vi "Tremor Interface.vi"() -> ()   [LabVIEW 2010]
uses:
  <vilib>/userDefined/High Color/IMAQdx.ctl
  Classes/Imported FFT Data.lvclass
  Controls/Interface states.ctl
  Classes/Waveform data.lvclass
  Classes/Video feed info.lvclass
  Controls/Timing Control.ctl
  Classes/Timer.lvclass
  <vilib>/Utility/xml.llb/Read From XML File(string).vi
  <vilib>/Analysis/2dsp.llb/1D Auto Correlation (DBL).vi
  <vilib>/Utility/xml.llb/Write to XML File(string).vi
  <vilib>/Utility/file.llb/Read From Spreadsheet File (string).vi
  <vilib>/Utility/file.llb/Read From Spreadsheet File (DBL).vi
  <vilib>/vision/NI_Vision_Development_Module.lvlib
  <vilib>/Analysis/NI_AAL_SigProc.lvlib
  <vilib>/Analysis/NI_AALBase.lvlib
  <vilib>/Analysis/NI_AALPro.lvlib
panel:
  in  "Reset spin":bool caption="Stop (F)"
  in  "spin control":bool caption="Stop (F)"
  in  "indicator radius":i16=10
  in  "indicator color":u32(colorbox)
  in  "speed":dbl=3.0
  in  "radius out":i16=130
  in  "camera feed":T1="cam0"
  in  "Circle width":i8(knob) scale=1.0..50.0
  in  "fill static indicator":bool
  in  "Circle style":T2(ring)
  in  "center color":u32(colorbox)
  in  "dot color":u32(colorbox)=782080
  out "Y Resolution":i32
  out "X Resolution":i32
  in  "Image Type":T3 items=["Grayscale (U8)", "Grayscale (I16)", "Grayscale (SGL)", "Complex (CSG)", "RGB (U32)", "HSL (U32)", "RGB (U64)", "Grayscale (U16)"]
  out "Frame Rate":dbl
  out "Image Number":u32
  in  "analyze (F3)":bool caption="Stop (F)"
  in  "record (F2)":bool caption="Stop (F)"
  in  "Save Config":bool caption="Stop (F)"
  in  "Optical FFTs":bool
  in  "Optical Data":bool
  out "number of channels":i32
  in  "Reset":bool caption="Stop (F)"
  in  "Quit":bool caption="Stop (F)"
  in  "camera (F1)":bool caption="Stop (F)"
  in  "Tab Control":T4(tab)
  out "Testing area":picture
  out "distance":dbl[](graph)
  out "distance":dbl
  out "angles":dbl[](graph)
  out "angles":dbl
  out "outside":bool
  out "Time outside circles":string
  out "outer counter":i8
  out "exterior":bool
  out "Time in exterior circle":string
  out "exterior counter":i8
  out "middle":bool
  out "Time in middle circle":string
  out "middle counter":i8
  out "interior":bool
  out "Time in inner circle":string
  out "inner counter":i8
  in  "Reset times":bool caption="Stop (F)"
  out "raw display":T5(plugin-control)
  in  "exterior color":u32(colorbox)=16711680
  in  "exterior circle":i16(knob)=164 scale=196.0..215.6
  in  "middle color":u32(colorbox)=16711680
  in  "middle circle":i16(knob)=93 scale=100.0..196.0
  in  "interior color":u32(colorbox)=16711680
  in  "interior circle":i16(knob)=57 scale=50.0..156.0
  in  "Rewind":bool
  in  "Forward":bool
  in  "Play/Stop":bool
  in  "Load file":bool
  in  "Video feed tab control":enum32{"Data", "Video controls"}(tab)
  out "displacement - vp":dbl[][](graph) caption="displacement"
  out "angles - vp":dbl[][](graph) caption="polar angles"
  out "angle (degrees) - vp":dbl caption="angle (degrees)"
  out "displacement - vp":dbl caption="displacement" format="%.2f"
  in  "Max Radius - video player":sgl=12.0 caption="Max Radius"
  in  "Min Radius - video player":sgl=2.0 caption="Min Radius"
  in  "Recording filter control 2":T6(tab)
  in  "Range - video player":cluster{"Lower value":sgl, "Upper value":sgl}={"Lower value"=250.0, "Upper value"=255.0} caption="Range"
  in  "Keep/Replace - video player":bool caption="Keep/Replace Value"
  in  "Replace Value - video player":sgl=1.0 caption="Replace Value" format="%.2f"
  in  "Toggle Controls - video player":T7={"Remove Border"=TRUE, "Fill Hole"=FALSE, "Remove Particles"=TRUE, "Particle Filter"=FALSE} caption="Toggle Controls"
  in  "Connectivity 4/8: 4":bool=TRUE
  in  "Connectivity 4/8: 5":bool=TRUE
  in  "Connectivity 4/8: 6":bool=TRUE
  in  "Keep/Remove Particles - video player":bool caption="Keep/Remove Particles"
  in  "Low Pass/High Pass: video player":bool caption="Low Pass/High Pass"
  in  "Number of Erosion: video player":i32=2 caption="Number of Erosions"
  in  "Square/Hexagon: video player":bool=TRUE caption="Square/Hexagon"
  in  "ROI Descriptor - video player":T8 caption="ROI Descriptor" {"Contours"."Type" items=["No Selection", "Point", "Line", "Rectangle", "Oval", "Polygon", "Freehand Region", "Annulus", "Unused2", "Unused3", "Broken Line", "Freehand Line", "Rotated Rectangle"]}
  in  "Selection Values - video player":T10(array[cluster]) caption="Selection Values" {"Measurement Parameter" items=["Center of Mass X", "Center of Mass Y", "First Pixel X", "First Pixel Y", "Bounding Rect Left", "Bounding Rect Top", "Bounding Rect Right", "Bounding Rect Bottom", "Max Feret Diameter Start X", "Max Feret Diameter Start Y", "Max Feret Diameter End X", "Max Feret Diameter End Y", "Max Horiz. Segment Length Left", "Max Horiz. Segment Length Right", "Max Horiz. Segment Length Row", "-", "Bounding Rect Width", "Bounding Rect Height", "Bounding Rect Diagonal", "Perimeter", "Convex Hull Perimeter", "Holes' Perimeter", "Max Feret Diameter", "Equivalent Ellipse Major Axis", "Equivalent Ellipse Minor Axis", "Equivalent Ellipse Minor Axis (Feret)", "Equivalent Rect Long Side", "Equivalent Rect Short Side", "Equivalent Rect Diagonal", "Equivalent Rect Short Side (Feret)", "Average Horiz. Segment Length", "Average Vert. Segment Length", "Hydraulic Radius", "Waddel Disk Diameter", "-", "Area", "Holes' Area", "Particle & Holes' Area", "Convex Hull Area", "Image Area", "-", "Number of Holes", "Number of Horiz. Segments", "Number of Vert. Segments", "-", "Orientation", "Max Feret Diameter Orientation", "-", "% Area/Image Area", "% Area/(Particle & Holes' Area)", "Ratio of Equivalent Ellipse Axes", "Ratio of Equivalent Rect Sides", "-", "Elongation Factor", "Compactness Factor", "Heywood Circularity Factor", "Type Factor", "-", "Sum X", "Sum Y", "Sum XX", "Sum XY", "Sum YY", "Sum XXX", "Sum XXY", "Sum XYY", "Sum YYY", "-", "Moment of Inertia XX", "Moment of Inertia XY", "Moment of Inertia YY", "Moment of Inertia XXX", "Moment of Inertia XXY", "Moment of Inertia XYY", "Moment of Inertia YYY", "Norm. Moment of Inertia XX", "Norm. Moment of Inertia XY", "Norm. Moment of Inertia YY", "Norm. Moment of Inertia XXX", "Norm. Moment of Inertia XXY", "Norm. Moment of Inertia XYY", "Norm. Moment of Inertia YYY", "Hu Moment 1", "Hu Moment 2", "Hu Moment 3", "Hu Moment 4", "Hu Moment 5", "Hu Moment 6", "Hu Moment 7"]; "Range Lower Value" format="%.2f"; "Range Upper Value" format="%.2f"}
  out "FPS":u32
  out "width":u32
  out "height":u32
  out "Number of Frames":u32
  out "Image video":T3 items=["Grayscale (U8)", "Grayscale (I16)", "Grayscale (SGL)", "Complex (CSG)", "RGB (U32)", "HSL (U32)", "RGB (U64)", "Grayscale (U16)"]
  in  "file path":path
  out "Image":T5(plugin-control)
  in  "Slide":cluster{u32, u32, u32}(slide) scale=-1.0..300.0
  in  "Recording filter control":T6(tab)
  in  "Range":cluster{"Lower value":sgl, "Upper value":sgl}={"Lower value"=250.0, "Upper value"=255.0}
  in  "Keep/Replace":bool caption="Keep/Replace Value"
  in  "Replace Value":sgl=1.0 format="%.2f"
  in  "Toggle Controls":T7={"Remove Border"=TRUE, "Fill Hole"=FALSE, "Remove Particles"=TRUE, "Particle Filter"=FALSE}
  in  "Connectivity 4/8: 2":bool=TRUE
  in  "Connectivity 4/8: 3":bool=TRUE
  in  "Keep/Remove Particles":bool
  in  "Connectivity 4/8:":bool=TRUE
  in  "Low Pass/High Pass:":bool
  in  "Number of Erosion:":i32=2
  in  "Square/Hexagon:":bool=TRUE
  in  "ROI Descriptor":T8 {"Contours"."Type" items=["No Selection", "Point", "Line", "Rectangle", "Oval", "Polygon", "Freehand Region", "Annulus", "Unused2", "Unused3", "Broken Line", "Freehand Line", "Rotated Rectangle"]}
  in  "Selection Values":T10(array[cluster]) {"Measurement Parameter" items=["Center of Mass X", "Center of Mass Y", "First Pixel X", "First Pixel Y", "Bounding Rect Left", "Bounding Rect Top", "Bounding Rect Right", "Bounding Rect Bottom", "Max Feret Diameter Start X", "Max Feret Diameter Start Y", "Max Feret Diameter End X", "Max Feret Diameter End Y", "Max Horiz. Segment Length Left", "Max Horiz. Segment Length Right", "Max Horiz. Segment Length Row", "-", "Bounding Rect Width", "Bounding Rect Height", "Bounding Rect Diagonal", "Perimeter", "Convex Hull Perimeter", "Holes' Perimeter", "Max Feret Diameter", "Equivalent Ellipse Major Axis", "Equivalent Ellipse Minor Axis", "Equivalent Ellipse Minor Axis (Feret)", "Equivalent Rect Long Side", "Equivalent Rect Short Side", "Equivalent Rect Diagonal", "Equivalent Rect Short Side (Feret)", "Average Horiz. Segment Length", "Average Vert. Segment Length", "Hydraulic Radius", "Waddel Disk Diameter", "-", "Area", "Holes' Area", "Particle & Holes' Area", "Convex Hull Area", "Image Area", "-", "Number of Holes", "Number of Horiz. Segments", "Number of Vert. Segments", "-", "Orientation", "Max Feret Diameter Orientation", "-", "% Area/Image Area", "% Area/(Particle & Holes' Area)", "Ratio of Equivalent Ellipse Axes", "Ratio of Equivalent Rect Sides", "-", "Elongation Factor", "Compactness Factor", "Heywood Circularity Factor", "Type Factor", "-", "Sum X", "Sum Y", "Sum XX", "Sum XY", "Sum YY", "Sum XXX", "Sum XXY", "Sum XYY", "Sum YYY", "-", "Moment of Inertia XX", "Moment of Inertia XY", "Moment of Inertia YY", "Moment of Inertia XXX", "Moment of Inertia XXY", "Moment of Inertia XYY", "Moment of Inertia YYY", "Norm. Moment of Inertia XX", "Norm. Moment of Inertia XY", "Norm. Moment of Inertia YY", "Norm. Moment of Inertia XXX", "Norm. Moment of Inertia XXY", "Norm. Moment of Inertia XYY", "Norm. Moment of Inertia YYY", "Hu Moment 1", "Hu Moment 2", "Hu Moment 3", "Hu Moment 4", "Hu Moment 5", "Hu Moment 6", "Hu Moment 7"]; "Range Lower Value" format="%.2f"; "Range Upper Value" format="%.2f"}
  out "Filtered Image":T5(plugin-control)
  out "Circles":T5(plugin-control)
  out "Circles Data":T11(array[cluster])
  in  "Max Radius":sgl=12.0
  in  "Min Radius":sgl=2.0
  out "autocorrelation theta":dbl[](graph)
  out "autocorrelation displacement":dbl[](graph)
  out "theta histogram":T12(graph)
  out "theta mean":dbl format="%0.2f"
  out "theta STD":dbl format="%0.2f"
  out "theta VAR":dbl format="%0.2f"
  out "FFT displacement":dbl[](graph)
  out "displacement histogram":T12(graph)
  out "displacement mean":dbl format="%0.2f"
  out "displacement STD":dbl format="%0.2f"
  out "displacement VAR":dbl format="%0.2f"
  out "FFT theta":dbl[](graph)
  out "FFT Visualizer":cluster{"Y":dbl[], "Y":dbl[]}[](graph)
  out "FFTs Table":string[][](table)
  in  "Add FFT?":bool
  in  "FFT Filename?":path=path "C:/Users/Justin Lee/Documents/LabVIEW Data"
  out "Peaks":string[][](table)
  in  "Percent (%)":dbl=10.0
  # "Feed Information"
  # "Indictator circle controls"
  # "Circle detection"
  # "Threshold controls"
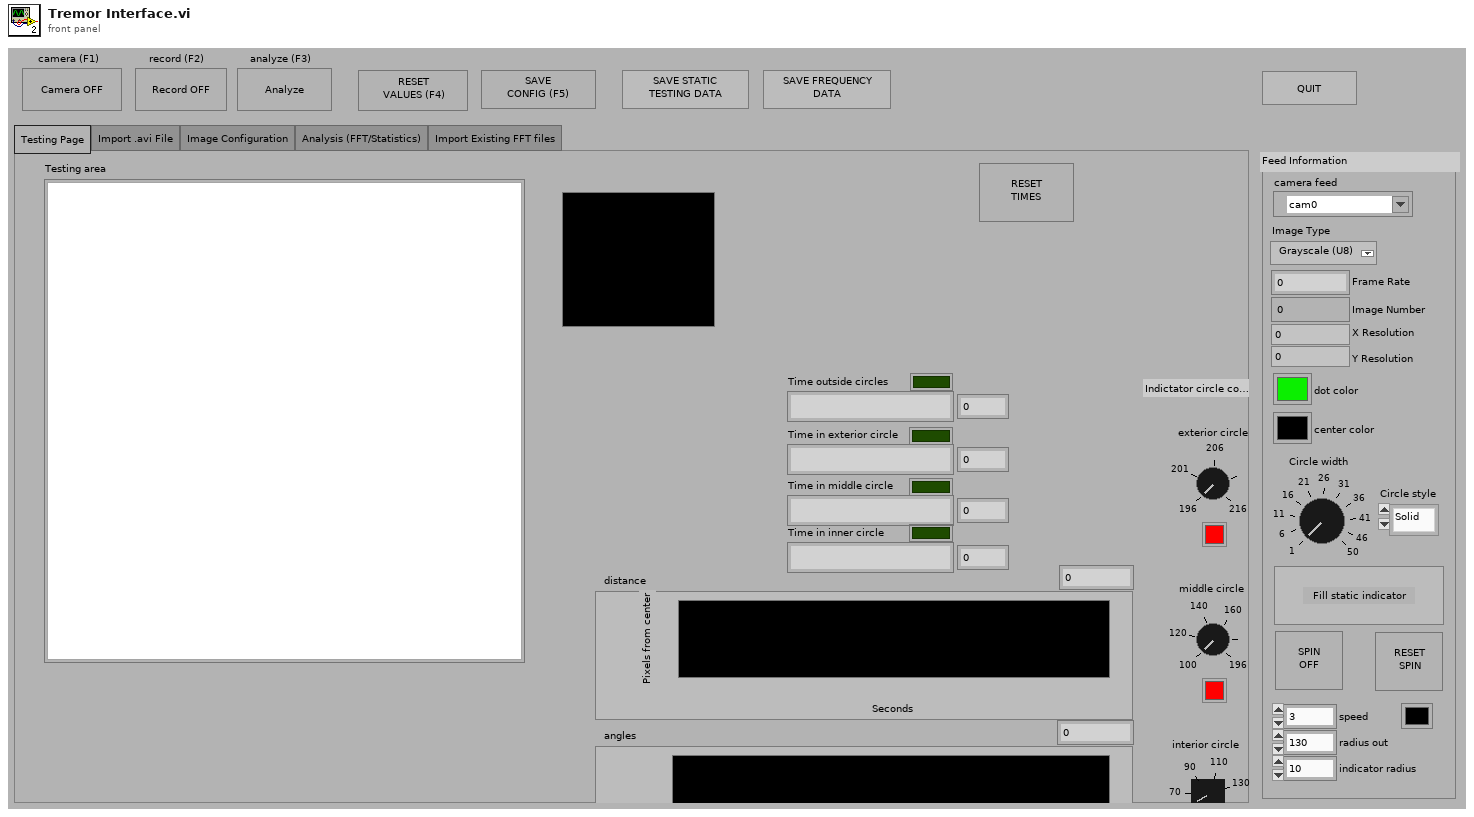
[diagram p1: front panel]
types:
  T1 = typedef "IMAQdx.ctl" = refnum<k21>
  T2 = enum32{"Solid", "Dash", "Dot", "DashDot", "DashDotDot"}
  T3 = typedef "Image Type" = u32
  T4 = enum32{"Testing Page", "Import .avi File", "Image Configuration", "Analysis (FFT/Statistics)", "Import Existing FFT files"}
  T5 = typedef "IMAQ Image.ctl" = refnum<image>
  T6 = enum32{"Threshold", "Toggle controls", "Particle connectivity", "ROI"}
  T7 = cluster{"Remove Border":bool, "Fill Hole":bool, "Remove Particles":bool, "Particle Filter":bool}
  T8 = typedef "ROI Descriptor" = cluster{"Global Rectangle":i32[], "Contours":cluster{"ID":enum32{"External", "Internal"}, "Type":u32, "Coordinates":i32[]}[]}
  T9 = typedef "Particle Parameters" = i32
  T10 = cluster{"Measurement Parameter":T9, "Range Lower Value":dbl, "Range Upper Value":dbl, "Range":bool, "Measurement Type":bool}[]
  T11 = cluster{"Pos. X":i32, "Pos. Y":i32, "Radius":i32, "Core Area":i32}[]
  T12 = cluster{"X Values":dbl[], "Histogram: h(x)":i32[]}
  T13 = cluster{"file path":path, "Replace Value - video player":sgl, "Keep/Replace - video player":bool, "Range - video player":cluster{"Lower value":sgl, "Upper value":sgl}, "Toggle Controls - video player":cluster{"Remove Border":bool, "Fill Hole":bool, "Remove Particles":bool, "Particle Filter":bool}, "Connectivity 4/8: 4":bool, "Connectivity 4/8: 5":bool, "Square/Hexagon: video player":bool, "Number of Erosion: video player":i32, "Low Pass/High Pass: video player":bool, cluster{"Global Rectangle":i32[], "Contours":cluster{"ID":enum32{"External", "Internal"}, "Type":u32, "Coordinates":i32[]}[]}, "Connectivity 4/8: 6":bool, "Selection Values - video player":cluster{"Measurement Parameter":T9, "Range Lower Value":dbl, "Range Upper Value":dbl, "Range":bool, "Measurement Type":bool}[], "Keep/Remove Particles - video player":bool, "Circle width":i8, "Circle style":enum32{"Solid", "Dash", "Dot", "DashDot", "DashDotDot"}, "fill static indicator":bool, "exterior color":u32, "middle color":u32, "interior color":u32, "exterior circle":i16, "middle circle":i16, "interior circle":i16, "center color":u32, "dot color":u32, "Max Radius - video player":sgl, "Min Radius - video player":sgl, "Replace Value":sgl, "Keep/Replace":bool, "Range":cluster{"Lower value":sgl, "Upper value":sgl}, u32, "Toggle Controls":cluster{"Remove Border":bool, "Fill Hole":bool, "Remove Particles":bool, "Particle Filter":bool}, "Connectivity 4/8: 3":bool, "Connectivity 4/8: 2":bool, "Square/Hexagon:":bool, "Number of Erosion:":i32, "Low Pass/High Pass:":bool, cluster{"Global Rectangle":i32[], "Contours":cluster{"ID":enum32{"External", "Internal"}, "Type":u32, "Coordinates":i32[]}[]}, "Connectivity 4/8:":bool, "Selection Values":cluster{"Measurement Parameter":T9, "Range Lower Value":dbl, "Range Upper Value":dbl, "Range":bool, "Measurement Type":bool}[], "Min Radius":sgl, "Max Radius":sgl, "Percent (%)":dbl, "FFT Filename?":path, "Keep/Remove Particles":bool}
  T14 = typedef "Interface states.ctl" = enum16{"Init", "Idle", "Record", "Reset", "Analyze", "Save", "Open - Analyze", "Watch"}
  T15 = cluster{"Global Rectangle":i32[], "Contours":cluster{"ID":enum32{"External", "Internal"}, "Type":u32, "Coordinates":i32[]}[]}
  T16 = enum16{"Load video", "Idle", "Play", "Rewind", "Forward", "Dispose"}
  T17 = typedef "Timing Control.ctl" = enum16{"Idle", "Start", "Continue", "Reset"}
  T18 = enum8{"Enabled", "Disabled", "Disabled and Grayed Out"}
  T19 = cluster{"Width":u16, "Style":enum32{"Solid", "Dash", "Dot", "DashDot", "DashDotDot"}}
  T20 = cluster{"Higher Cursor value":u32, "Lower Cursor value":u32, "Higher Cursor value":u32}
  T21 = cluster{"Circle width":i8, "Circle style":enum32{"Solid", "Dash", "Dot", "DashDot", "DashDotDot"}}
  T22 = cluster{"Circle width":i8, "Style":enum32{"Solid", "Dash", "Dot", "DashDot", "DashDotDot"}}
  T23 = typedef "LVBoundsTypeDef.ctl" = cluster{"Width":u32, "Height":u32}
  T24 = cluster{"Value":path, "Value":sgl, "Value":bool, "Value":cluster{"Lower value":sgl, "Upper value":sgl}, "Value":cluster{"Remove Border":bool, "Fill Hole":bool, "Remove Particles":bool, "Particle Filter":bool}, "Value":bool, "Value":bool, "Value":bool, "Value":i32, "Value":bool, "Value":cluster{"Global Rectangle":i32[], "Contours":cluster{"ID":enum32{"External", "Internal"}, "Type":u32, "Coordinates":i32[]}[]}, "Value":bool, "Value":cluster{"Measurement Parameter":T9, "Range Lower Value":dbl, "Range Upper Value":dbl, "Range":bool, "Measurement Type":bool}[], "Value":bool, "Value":i8, "Value":enum32{"Solid", "Dash", "Dot", "DashDot", "DashDotDot"}, "Value":bool, "Value":u32, "Value":u32, "Value":u32, "Value":i16, "Value":i16, "Value":i16, "Value":u32, "Value":u32, "Value":sgl, "Value":sgl, "Value":sgl, "Value":bool, "Value":cluster{"Lower value":sgl, "Upper value":sgl}, "Value":u32, "Value":cluster{"Remove Border":bool, "Fill Hole":bool, "Remove Particles":bool, "Particle Filter":bool}, "Value":bool, "Value":bool, "Value":bool, "Value":i32, "Value":bool, "Value":cluster{"Global Rectangle":i32[], "Contours":cluster{"ID":enum32{"External", "Internal"}, "Type":u32, "Coordinates":i32[]}[]}, "Value":bool, "Value":cluster{"Measurement Parameter":T9, "Range Lower Value":dbl, "Range Upper Value":dbl, "Range":bool, "Measurement Type":bool}[], "Value":sgl, "Value":sgl, "Value":dbl, "Value":path, "Value":bool}
  T25 = typedef "LVPoint32TypeDef.ctl" = cluster{"Horizontal":i32, "Vertical":i32}
  T26 = typedef "LVRowAndColumnTypeDef.ctl" = cluster{"Row":i32, "Column":i32}
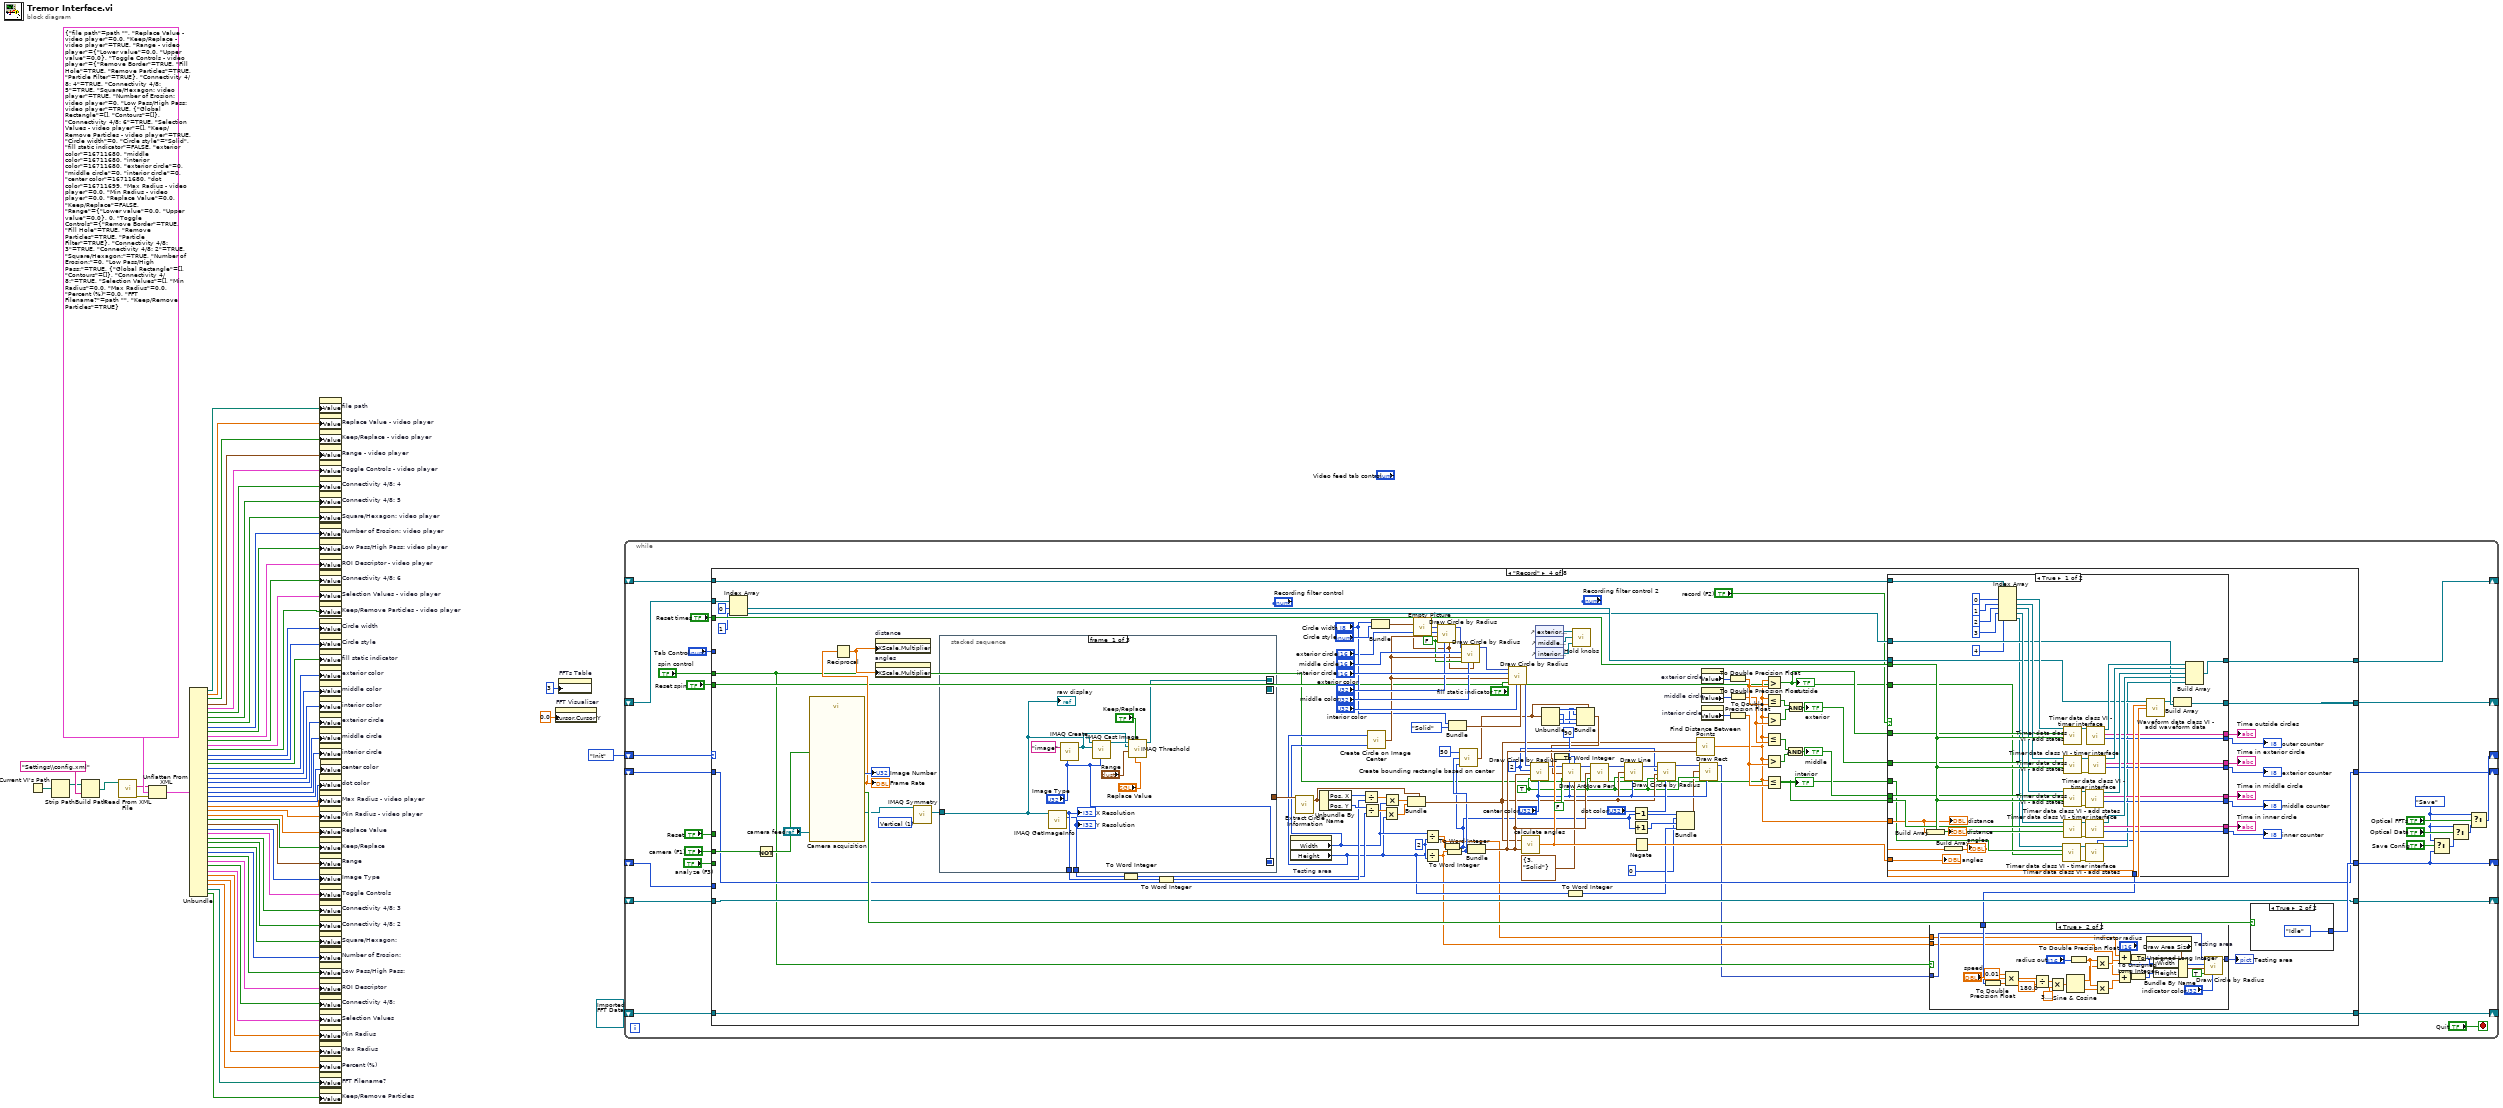
[diagram p0: block diagram]
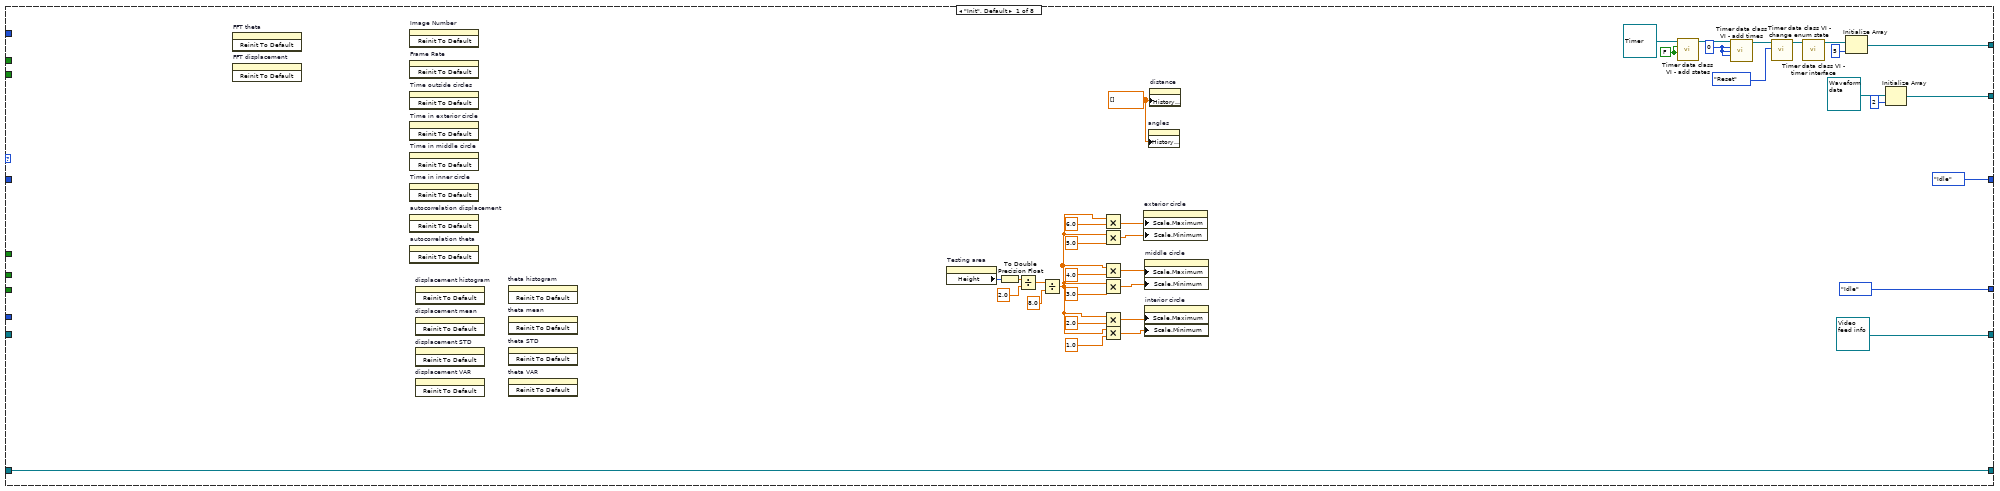
[diagram p2: hidden frame]
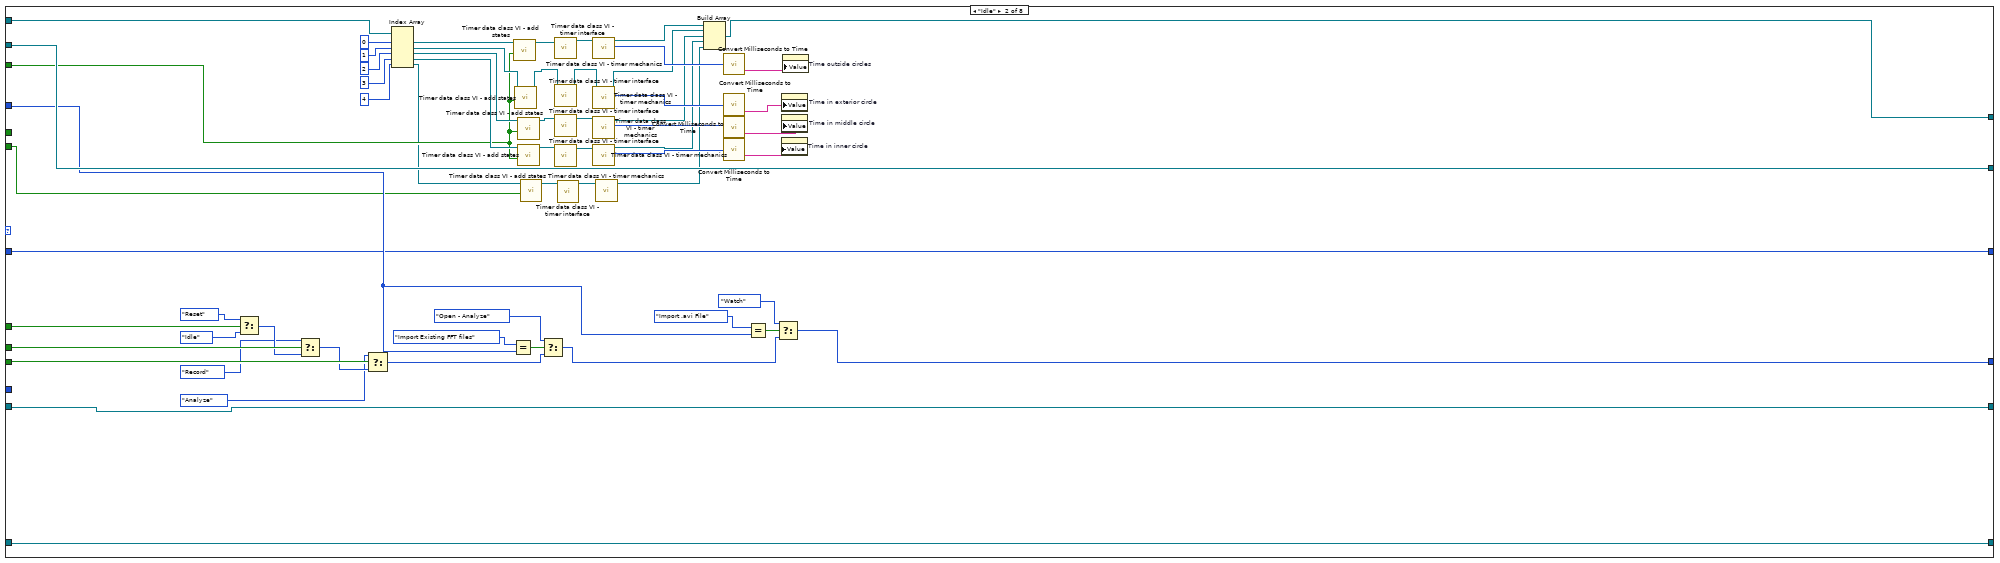
[diagram p3: hidden frame]
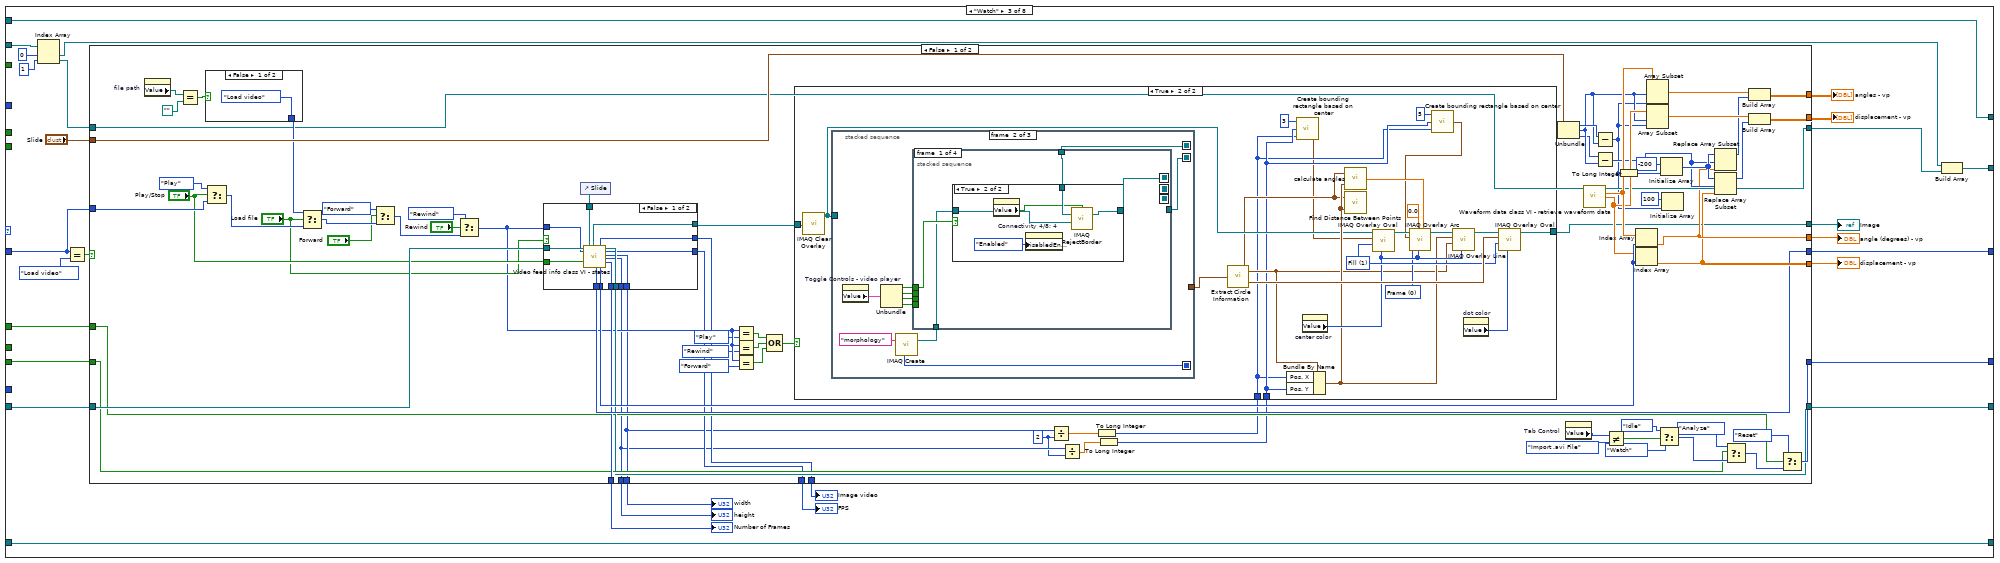
[diagram p4: hidden frame]
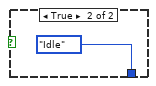
[diagram p5: hidden frame]
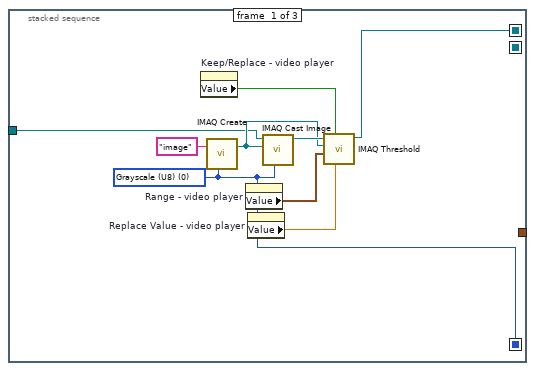
[diagram p7: hidden frame]
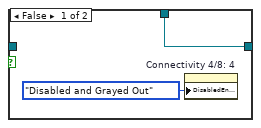
[diagram p8: hidden frame]
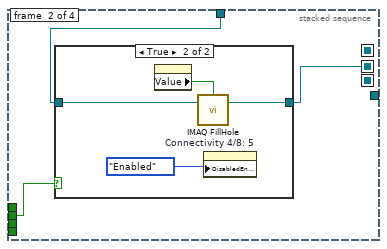
[diagram p9: hidden frame]
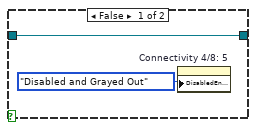
[diagram p10: hidden frame]
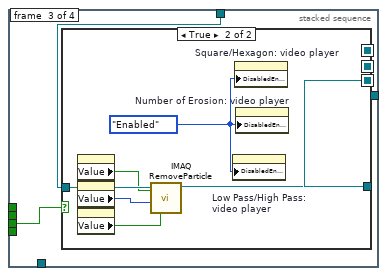
[diagram p11: hidden frame]
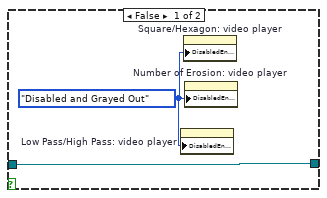
[diagram p12: hidden frame]
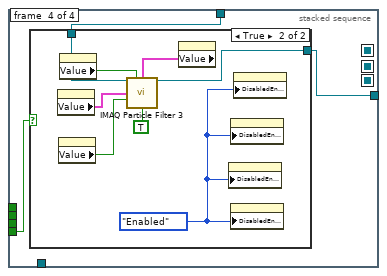
[diagram p13: hidden frame]
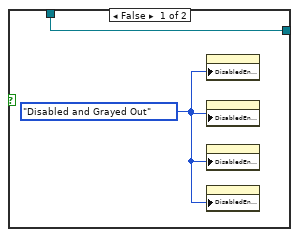
[diagram p14: hidden frame]
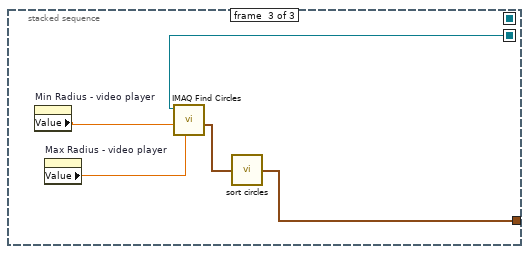
[diagram p15: hidden frame]
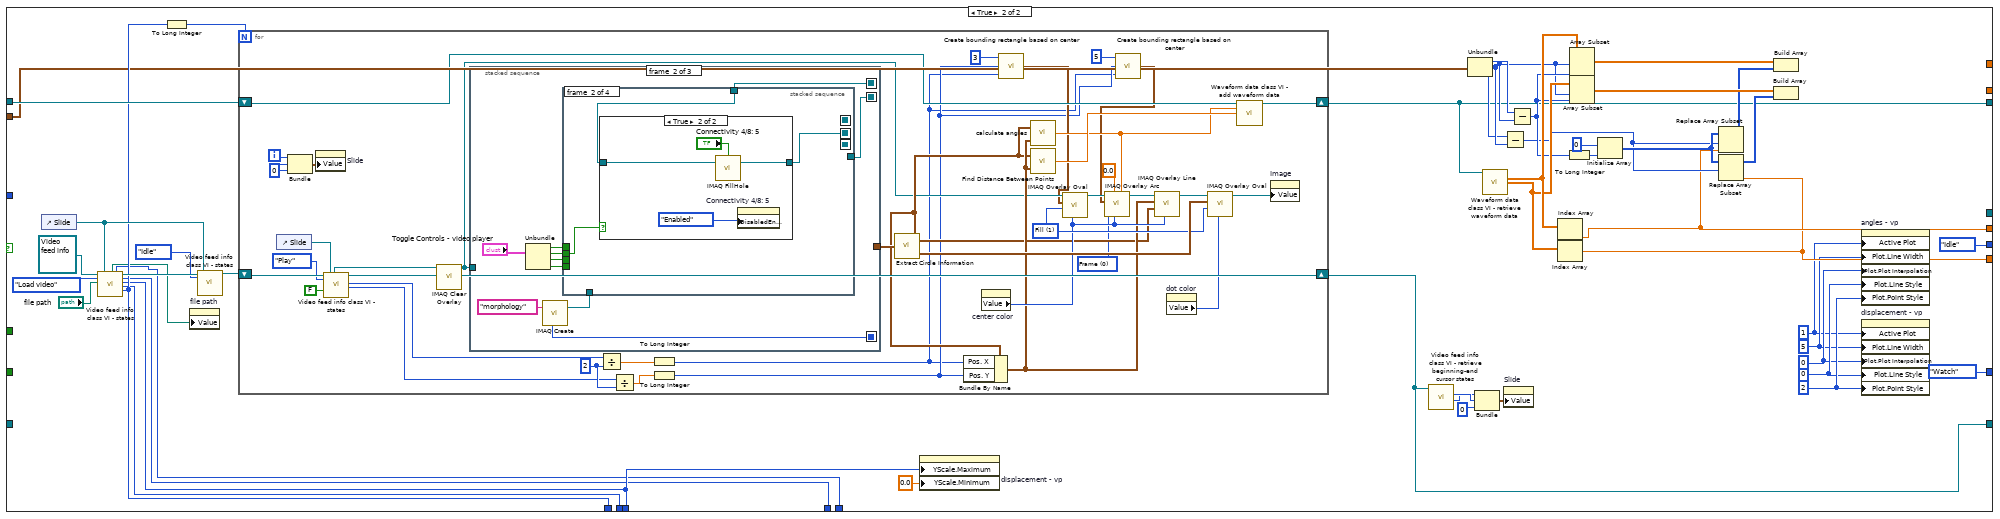
[diagram p17: hidden frame]
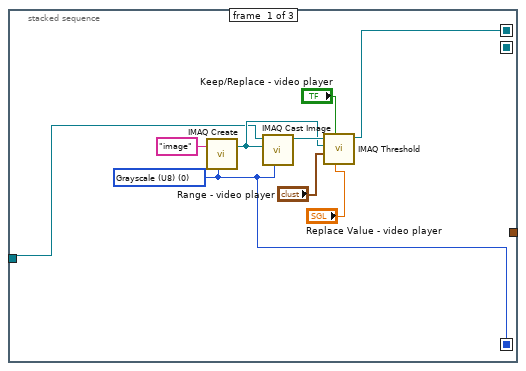
[diagram p18: hidden frame]
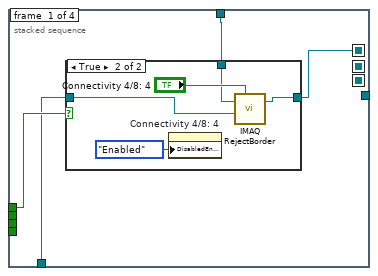
[diagram p19: hidden frame]
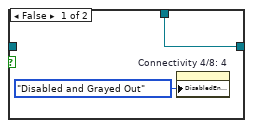
[diagram p20: hidden frame]
diagram:
  n1 = Current VI's Path() -> (path=w51:path)
  n2 = Strip Path(path=w51) -> (stripped path=w52:path)  [unwired: 1 out]
  n3 = Build Path(base path=w52, name or relative path="Settings\\config.xml") -> (appended path=w49:path)
  n4 = call-poly <vilib>:"Read From XML File.vi"("XML File Path"=w49) -> ("error out"=w50:errorcluster, "XML Elements"=w47:string)  [unwired: 8 in, 1 out]
  n5 = Unflatten From XML(xml string=w47, type=T13 {"file path"=path "", "Replace Value - video player"=0.0, "Keep/Replace - video player"=TRUE, "Range - video player"={"Lower value"=0.0, "Upper value"=0.0}, "Toggle Controls - video player"={"Remove Border"=TRUE, "Fill Hole"=TRUE, "Remove Particles"=TRUE, "Particle Filter"=TRUE}, "Connectivity 4/8: 4"=TRUE, "Connectivity 4/8: 5"=TRUE, "Square/Hexagon: video player"=TRUE, "Number of Erosion: video player"=0, "Low Pass/High Pass: video player"=TRUE, {"Global Rectangle"=[], "Contours"=[]}, "Connectivity 4/8: 6"=TRUE, "Selection Values - video player"=[], "Keep/Remove Particles - video player"=TRUE, "Circle width"=0, "Circle style"=enum."Solid", "fill static indicator"=FALSE, "exterior color"=16711680, "middle color"=16711680, "interior color"=16711680, "exterior circle"=0, "middle circle"=0, "interior circle"=0, "center color"=16711680, "dot color"=16711699, "Max Radius - video player"=0.0, "Min Radius - video player"=0.0, "Replace Value"=0.0, "Keep/Replace"=FALSE, "Range"={"Lower value"=0.0, "Upper value"=0.0}, 0, "Toggle Controls"={"Remove Border"=TRUE, "Fill Hole"=TRUE, "Remove Particles"=TRUE, "Particle Filter"=TRUE}, "Connectivity 4/8: 3"=TRUE, "Connectivity 4/8: 2"=TRUE, "Square/Hexagon:"=TRUE, "Number of Erosion:"=0, "Low Pass/High Pass:"=TRUE, {"Global Rectangle"=[], "Contours"=[]}, "Connectivity 4/8:"=TRUE, "Selection Values"=[], "Min Radius"=0.0, "Max Radius"=0.0, "Percent (%)"=0.0, "FFT Filename?"=path "", "Keep/Remove Particles"=TRUE}, error in (no error)=w50) -> (value=w46:T13)  [unwired: 1 out]
  n6 = Unbundle(w46) -> ("file path"=w45:path, "Replace Value - video player"=w44:sgl, "Keep/Replace - video player"=w43:bool, "Range - video player"=w42:cluster{"Lower value":sgl, "Upper value":sgl}, "Toggle Controls - video player"=w41:T7, "Connectivity 4/8: 4"=w40:bool, "Connectivity 4/8: 5"=w39:bool, "Square/Hexagon: video player"=w38:bool, "Number of Erosion: video player"=w37:i32, "Low Pass/High Pass: video player"=w36:bool, w35:T15, "Connectivity 4/8: 6"=w34:bool, "Selection Values - video player"=w33:T10, "Keep/Remove Particles - video player"=w32:bool, "Circle width"=w31:i8, "Circle style"=w30:T2, "fill static indicator"=w29:bool, "exterior color"=w1:u32, "middle color"=w2:u32, "interior color"=w3:u32, "exterior circle"=w4:i16, "middle circle"=w5:i16, "interior circle"=w6:i16, "center color"=w7:u32, "dot color"=w8:u32, "Max Radius - video player"=w9:sgl, "Min Radius - video player"=w10:sgl, "Replace Value"=w11:sgl, "Keep/Replace"=w12:bool, "Range"=w13:cluster{"Lower value":sgl, "Upper value":sgl}, w14:u32, "Toggle Controls"=w15:T7, "Connectivity 4/8: 3"=w16:bool, "Connectivity 4/8: 2"=w17:bool, "Square/Hexagon:"=w18:bool, "Number of Erosion:"=w19:i32, "Low Pass/High Pass:"=w20:bool, w21:T15, "Connectivity 4/8:"=w22:bool, "Selection Values"=w23:T10, "Min Radius"=w24:sgl, "Max Radius"=w25:sgl, "Percent (%)"=w26:dbl, "FFT Filename?"=w27:path, "Keep/Remove Particles"=w28:bool)
  n7 = property on="file path" class="Path"("Value"=w45) -> ()  [unwired: 2 in, 2 out]
  n8 = property on="Replace Value - video player" class="DigNum (strict)"("Value"=w44) -> ()  [unwired: 2 in, 2 out]
  n9 = property on="Keep/Replace - video player" class="Bool (strict)"("Value"=w43) -> ()  [unwired: 2 in, 2 out]
  n10 = property on="Range - video player" class="Clust (strict)"("Value"=w42) -> ()  [unwired: 2 in, 2 out]
  n11 = property on="Toggle Controls - video player" class="Clust (strict)"("Value"=w41) -> ()  [unwired: 2 in, 2 out]
  n12 = property on="Connectivity 4/8: 4" class="Bool (strict)"("Value"=w40) -> ()  [unwired: 2 in, 2 out]
  n13 = property on="Connectivity 4/8: 5" class="Bool (strict)"("Value"=w39) -> ()  [unwired: 2 in, 2 out]
  n14 = property on="Square/Hexagon: video player" class="Bool (strict)"("Value"=w38) -> ()  [unwired: 2 in, 2 out]
  n15 = property on="Number of Erosion: video player" class="DigNum (strict)"("Value"=w37) -> ()  [unwired: 2 in, 2 out]
  n16 = property on="Low Pass/High Pass: video player" class="Bool (strict)"("Value"=w36) -> ()  [unwired: 2 in, 2 out]
  n17 = property on="ROI Descriptor - video player" class="Clust (strict)"("Value"=w35) -> ()  [unwired: 2 in, 2 out]
  n18 = property on="Connectivity 4/8: 6" class="Bool (strict)"("Value"=w34) -> ()  [unwired: 2 in, 2 out]
  n19 = property on="Selection Values - video player" class="Arr (strict)"("Value"=w33) -> ()  [unwired: 2 in, 2 out]
  n20 = property on="Keep/Remove Particles - video player" class="Bool (strict)"("Value"=w32) -> ()  [unwired: 2 in, 2 out]
  n21 = property on="Circle width" class="Knob (strict)"("Value"=w31) -> ()  [unwired: 2 in, 2 out]
  n22 = property on="Circle style" class="Enum (strict)"("Value"=w30) -> ()  [unwired: 2 in, 2 out]
  n23 = property on="fill static indicator" class="Bool (strict)"("Value"=w29) -> ()  [unwired: 2 in, 2 out]
  n24 = property on="exterior color" class="ColBox"("Value"=w1) -> ()  [unwired: 2 in, 2 out]
  n25 = property on="middle color" class="ColBox"("Value"=w2) -> ()  [unwired: 2 in, 2 out]
  n26 = property on="interior color" class="ColBox"("Value"=w3) -> ()  [unwired: 2 in, 2 out]
  n27 = property on="exterior circle" class="Knob (strict)"("Value"=w4) -> ()  [unwired: 2 in, 2 out]
  n28 = property on="middle circle" class="Knob (strict)"("Value"=w5) -> ()  [unwired: 2 in, 2 out]
  n29 = property on="interior circle" class="Knob (strict)"("Value"=w6) -> ()  [unwired: 2 in, 2 out]
  n30 = property on="dot color" class="ColBox"("Value"=w8) -> ()  [unwired: 2 in, 2 out]
  n31 = property on="Max Radius - video player" class="DigNum (strict)"("Value"=w9) -> ()  [unwired: 2 in, 2 out]
  n32 = property on="Min Radius - video player" class="DigNum (strict)"("Value"=w10) -> ()  [unwired: 2 in, 2 out]
  n33 = property on="Replace Value" class="DigNum (strict)"("Value"=w11) -> ()  [unwired: 2 in, 2 out]
  n34 = property on="Keep/Replace" class="Bool (strict)"("Value"=w12) -> ()  [unwired: 2 in, 2 out]
  n35 = property on="Range" class="Clust (strict)"("Value"=w13) -> ()  [unwired: 2 in, 2 out]
  n36 = property on="Image Type" class="Ring (strict)"("Value"=w14) -> ()  [unwired: 2 in, 2 out]
  n37 = property on="Toggle Controls" class="Clust (strict)"("Value"=w15) -> ()  [unwired: 2 in, 2 out]
  n38 = property on="Connectivity 4/8: 3" class="Bool (strict)"("Value"=w16) -> ()  [unwired: 2 in, 2 out]
  n39 = property on="Connectivity 4/8: 2" class="Bool (strict)"("Value"=w17) -> ()  [unwired: 2 in, 2 out]
  n40 = property on="Square/Hexagon:" class="Bool (strict)"("Value"=w18) -> ()  [unwired: 2 in, 2 out]
  n41 = property on="Number of Erosion:" class="DigNum (strict)"("Value"=w19) -> ()  [unwired: 2 in, 2 out]
  n42 = property on="Low Pass/High Pass:" class="Bool (strict)"("Value"=w20) -> ()  [unwired: 2 in, 2 out]
  n43 = property on="ROI Descriptor" class="Clust (strict)"("Value"=w21) -> ()  [unwired: 2 in, 2 out]
  n44 = property on="Connectivity 4/8:" class="Bool (strict)"("Value"=w22) -> ()  [unwired: 2 in, 2 out]
  n45 = property on="Selection Values" class="Arr (strict)"("Value"=w23) -> ()  [unwired: 2 in, 2 out]
  n46 = property on="Min Radius" class="DigNum (strict)"("Value"=w24) -> ()  [unwired: 2 in, 2 out]
  n47 = property on="Max Radius" class="DigNum (strict)"("Value"=w25) -> ()  [unwired: 2 in, 2 out]
  n48 = property on="Percent (%)" class="DigNum (strict)"("Value"=w26) -> ()  [unwired: 2 in, 2 out]
  n49 = property on="FFT Filename?" class="Path"("Value"=w27) -> ()  [unwired: 2 in, 2 out]
  n50 = property on="Keep/Remove Particles" class="Bool (strict)"("Value"=w28) -> ()  [unwired: 2 in, 2 out]
  n51 = property on="center color" class="ColBox"("Value"=w7) -> ()  [unwired: 2 in, 2 out]
  n52 = property on="FFT Visualizer" class="XYGraph (strict)"("Cursor.Cursor Y"=0.0 ("Cursor.Cursor Position:Cursor Y")) -> ()  [unwired: 2 in, 2 out]
  n53 = property on="FFTs Table" class="Tbl (strict)"("Number of Columns"=u32 3) -> ()  [unwired: 2 in, 2 out]
  n54 = while {
    shift-right: [w77] -> _
    shift-left: Interface_states."Init" ("Enum") -> [w85]
    shift-right: [w80] -> _
    shift-left: _ -> [w81]
    shift-right: [w62] -> _
    shift-left: _ -> [w75]
    shift-right: [w73] -> _
    shift-left: _ -> [w74]
    shift-right: [w69] -> _
    shift-left: refnum<class "Imported FFT Data.lvclass"> refnum ("Imported FFT Data.lvclass") -> [w70]
    shift-right: [w68] -> _
    shift-left: _ -> [w67]
    shift-right: [w66] -> _
    shift-left: _ -> [w65]
    stop <- "Quit" stop-if-true
    w61 = Interface_states."Save" ("Enum")
    n55 = case shown="\"Record\"" w85 {
      tunnel: "Reset" -> [_ w181 w189 _ _ _ _ _]
      tunnel: "camera (F1)" -> [_ w180 _ w662 _ _ _ _]
      tunnel: "analyze (F3)" -> [_ w179 w190 _ _ _ _ _]
      tunnel: [Interface_states."Idle" ("Enum") w132 w209 w659 Interface_states."Init" ("Enum") Interface_states."Idle" ("Enum") w942 w1117] -> w62
      tunnel: w81 -> [_ w176 w206 w617 w863 w900 w937 w1118]
      tunnel: [w106 w176 w183 w612 w863 w891 w937 w1118] -> w80
      tunnel: w75 -> [_ _ _ _ _ _ w942 _]
      tunnel: w74 -> [_ w151 w210 w658 w862 w904 w933 w1119]
      tunnel: [w118 w150 w210 w657 w862 w904 w933 w1119] -> w73
      tunnel: "Reset times" -> [_ w145 _ w656 _ _ _ _]
      tunnel: "Tab Control" -> [_ w135 _ _ _ w887 w935 _]
      tunnel: w70 -> [w112 w142 w182 w655 w861 w903 w941 w1116]
      tunnel: [w112 w142 w182 w655 w861 w903 w941 w1115] -> w69
      tunnel: w67 -> [_ w131 w208 w654 w859 w899 w940 w1114]
      tunnel: [refnum<class "Video feed info.lvclass"> refnum ("Video feed info.lvclass") w131 w204 w654 w859 w899 w940 w1114] -> w68
      tunnel: [T16."Idle" ("States") w130 w203 w653 w858 w898 w939 w1113] -> w66
      tunnel: w65 -> [_ w130 w194 w653 w858 w898 w939 w1113]
      tunnel: "Reset spin" -> [_ w126 _ w550 _ _ _ _]
      tunnel: "spin control" -> [_ _ _ w547 _ _ _ _]
      frame "Init", Default {
        w104 = dbl[] [] ("History Data")
        w115 = FALSE ("Reset")
        w120 = u32 0 ("Milliseconds")
        n56 = invoke on="FFT theta" class="WFGraph (strict)" method="Reinit To Default"() -> ()  [unwired: 3 in, 3 out]
        n57 = invoke on="FFT displacement" class="WFGraph (strict)" method="Reinit To Default"() -> ()  [unwired: 3 in, 3 out]
        n58 = invoke on="Image Number" class="DigNum (strict)" method="Reinit To Default"() -> ()  [unwired: 3 in, 3 out]
        n59 = invoke on="Frame Rate" class="DigNum (strict)" method="Reinit To Default"() -> ()  [unwired: 3 in, 3 out]
        n60 = invoke on="Time outside circles" class="Str" method="Reinit To Default"() -> ()  [unwired: 3 in, 3 out]
        n61 = invoke on="Time in exterior circle" class="Str" method="Reinit To Default"() -> ()  [unwired: 3 in, 3 out]
        n62 = invoke on="Time in middle circle" class="Str" method="Reinit To Default"() -> ()  [unwired: 3 in, 3 out]
        n63 = invoke on="Time in inner circle" class="Str" method="Reinit To Default"() -> ()  [unwired: 3 in, 3 out]
        n64 = invoke on="autocorrelation displacement" class="WFGraph (strict)" method="Reinit To Default"() -> ()  [unwired: 3 in, 3 out]
        n65 = invoke on="autocorrelation theta" class="WFGraph (strict)" method="Reinit To Default"() -> ()  [unwired: 3 in, 3 out]
        n66 = invoke on="displacement histogram" class="XYGraph (strict)" method="Reinit To Default"() -> ()  [unwired: 3 in, 3 out]
        n67 = invoke on="displacement mean" class="DigNum (strict)" method="Reinit To Default"() -> ()  [unwired: 3 in, 3 out]
        n68 = invoke on="displacement STD" class="DigNum (strict)" method="Reinit To Default"() -> ()  [unwired: 3 in, 3 out]
        n69 = invoke on="displacement VAR" class="DigNum (strict)" method="Reinit To Default"() -> ()  [unwired: 3 in, 3 out]
        n70 = invoke on="theta histogram" class="XYGraph (strict)" method="Reinit To Default"() -> ()  [unwired: 3 in, 3 out]
        n71 = invoke on="theta mean" class="DigNum (strict)" method="Reinit To Default"() -> ()  [unwired: 3 in, 3 out]
        n72 = invoke on="theta STD" class="DigNum (strict)" method="Reinit To Default"() -> ()  [unwired: 3 in, 3 out]
        n73 = invoke on="theta VAR" class="DigNum (strict)" method="Reinit To Default"() -> ()  [unwired: 3 in, 3 out]
        n74 = property on="Testing area" class="Pict"() -> ("Height"=w103:u32)  [unwired: 2 in, 2 out]
        n75 = To Double Precision Float(number=w103) -> (double precision float=w102:dbl)
        n76 = Divide(x=w102, y=2.0) -> (x/y=w100:dbl)
        n77 = Divide(x=w100, y=8.0) -> (x/y=w93:dbl)
        n78 = Multiply(x=w93, y=6.0) -> (x*y=w87:dbl)
        n79 = Multiply(x=w93, y=5.0) -> (x*y=w88:dbl)
        n80 = Multiply(x=w93, y=4.0) -> (x*y=w98:dbl)
        n81 = Multiply(x=w93, y=3.0) -> (x*y=w97:dbl)
        n82 = Multiply(x=w93, y=2.0) -> (x*y=w90:dbl)
        n83 = Multiply(x=w93, y=1.0) -> (x*y=w89:dbl)
        n84 = property on="exterior circle" class="Knob (strict)"("Scale.Maximum"=w87, "Scale.Minimum"=w88) -> ()  [unwired: 2 in, 2 out]
        n85 = property on="middle circle" class="Knob (strict)"("Scale.Maximum"=w98, "Scale.Minimum"=w97) -> ()  [unwired: 2 in, 2 out]
        n86 = property on="interior circle" class="Knob (strict)"("Scale.Maximum"=w90, "Scale.Minimum"=w89) -> ()  [unwired: 2 in, 2 out]
        n87 = property on="angles" class="WFChart (strict)"("History Data"=w104) -> ()  [unwired: 2 in, 2 out]
        n88 = property on="distance" class="WFChart (strict)"("History Data"=w104) -> ()  [unwired: 2 in, 2 out]
        n89 = call-dynamic "Timer data class VI - add states.vi"("Reset"=w115, "Start/Stop"=w115, "Timer in"=refnum<class "Timer.lvclass"> refnum ("Timer.lvclass")) -> ("Timer out"=w121:refnum<class "Timer.lvclass">)  [unwired: 7 in, 1 out]
        n90 = call-dynamic "Timer data class VI - add times.vi"("Timer in"=w121, "Milliseconds"=w120, "Time 1"=w120, "Time 2"=w120) -> ("Timer out"=w117:refnum<class "Timer.lvclass">)  [unwired: 10 in, 1 out]
        n91 = call-dynamic "Timer data class VI - change enum state.vi"("State"=Timing_Control."Reset", "Timer in"=w117) -> ("Timer out"=w114:refnum<class "Timer.lvclass">)  [unwired: 8 in, 1 out]
        n92 = call-dynamic "Timer data class VI - timer interface.vi"("Timer in"=w114) -> ("Timer out"=w113:refnum<class "Timer.lvclass">)  [unwired: 6 in, 4 out]
        n93 = Initialize Array(w113, 5 ("dimension size")) -> (w118:refnum<class "Timer.lvclass">[])
        n94 = Initialize Array(refnum<class "Waveform data.lvclass"> refnum ("Waveform data.lvclass"), 2 ("dimension size")) -> (w106:refnum<class "Waveform data.lvclass">[])
      }
      frame "Idle" {
        n95 = Select(t=Interface_states."Reset" ("Enum"), s=w181, f=Interface_states."Idle" ("Enum")) -> (s? t:f=w178:T14)
        n96 = Select(t=Interface_states."Record" ("Enum"), s=w180, f=w178) -> (s? t:f=w177:T14)
        n97 = Select(t=Interface_states."Analyze" ("Enum"), s=w179, f=w177) -> (s? t:f=w143:T14)
        n98 = Index Array(array=w151, index #1=0 ("index"), index #2=1 ("index"), index #3=2 ("index"), index #4=3 ("index"), index #5=4 ("index")) -> (element #1=w171:refnum<class "Timer.lvclass">, element #2=w170:refnum<class "Timer.lvclass">, element #3=w169:refnum<class "Timer.lvclass">, element #4=w168:refnum<class "Timer.lvclass">, element #5=w125:refnum<class "Timer.lvclass">)
        n99 = Equal?(x=T4."Import Existing FFT files", y=w135) -> (x = y?=w144:bool)
        n100 = call-dynamic "Timer data class VI - add states.vi"("Reset"=w145, "Timer in"=w171) -> ("Timer out"=w159:refnum<class "Timer.lvclass">)  [unwired: 8 in, 1 out]
        n101 = call-dynamic "Timer data class VI - add states.vi"("Reset"=w145, "Timer in"=w170) -> ("Timer out"=w157:refnum<class "Timer.lvclass">)  [unwired: 8 in, 1 out]
        n102 = call-dynamic "Timer data class VI - add states.vi"("Reset"=w145, "Timer in"=w169) -> ("Timer out"=w155:refnum<class "Timer.lvclass">)  [unwired: 8 in, 1 out]
        n103 = call-dynamic "Timer data class VI - add states.vi"("Reset"=w145, "Timer in"=w168) -> ("Timer out"=w153:refnum<class "Timer.lvclass">)  [unwired: 8 in, 1 out]
        n104 = call-dynamic "Timer data class VI - add states.vi"("Reset"=w126, "Timer in"=w125) -> ("Timer out"=w124:refnum<class "Timer.lvclass">)  [unwired: 8 in, 1 out]
        n105 = Select(t=Interface_states."Open - Analyze" ("Enum"), s=w144, f=w143) -> (s? t:f=w133:T14)
        n106 = call-dynamic "Timer data class VI - timer interface.vi"("Timer in"=w159) -> ("Timer out"=w158:refnum<class "Timer.lvclass">)  [unwired: 6 in, 4 out]
        n107 = call-dynamic "Timer data class VI - timer interface.vi"("Timer in"=w157) -> ("Timer out"=w156:refnum<class "Timer.lvclass">)  [unwired: 6 in, 4 out]
        n108 = call-dynamic "Timer data class VI - timer interface.vi"("Timer in"=w155) -> ("Timer out"=w154:refnum<class "Timer.lvclass">)  [unwired: 6 in, 4 out]
        n109 = call-dynamic "Timer data class VI - timer interface.vi"("Timer in"=w153) -> ("Timer out"=w152:refnum<class "Timer.lvclass">)  [unwired: 6 in, 4 out]
        n110 = call-dynamic "Timer data class VI - timer interface.vi"("Timer in"=w124) -> ("Timer out"=w123:refnum<class "Timer.lvclass">)  [unwired: 6 in, 4 out]
        n111 = call-dynamic "Timer data class VI - timer mechanics.vi"("Timer in"=w158) -> ("elapsed time (milliseconds)"=w167:u32, "Timer out"=w163:refnum<class "Timer.lvclass">)  [unwired: 8 in, 1 out]
        n112 = call-dynamic "Timer data class VI - timer mechanics.vi"("Timer in"=w156) -> ("elapsed time (milliseconds)"=w166:u32, "Timer out"=w162:refnum<class "Timer.lvclass">)  [unwired: 8 in, 1 out]
        n113 = call-dynamic "Timer data class VI - timer mechanics.vi"("Timer in"=w154) -> ("elapsed time (milliseconds)"=w165:u32, "Timer out"=w161:refnum<class "Timer.lvclass">)  [unwired: 8 in, 1 out]
        n114 = call-dynamic "Timer data class VI - timer mechanics.vi"("Timer in"=w152) -> ("elapsed time (milliseconds)"=w164:u32, "Timer out"=w160:refnum<class "Timer.lvclass">)  [unwired: 8 in, 1 out]
        n115 = call-dynamic "Timer data class VI - timer mechanics.vi"("Timer in"=w123) -> ("Timer out"=w122:refnum<class "Timer.lvclass">)  [unwired: 8 in, 2 out]
        n116 = Build Array(w163, w162, w161, w160, w122) -> (w150:refnum<class "Timer.lvclass">[])
        n117 = call "Convert Milliseconds to Time.vi"("milliseconds"=w167) -> ("elapsed time"=w149:string)  [unwired: 1 in]
        n118 = call "Convert Milliseconds to Time.vi"("milliseconds"=w166) -> ("elapsed time"=w148:string)  [unwired: 1 in]
        n119 = call "Convert Milliseconds to Time.vi"("milliseconds"=w165) -> ("elapsed time"=w147:string)  [unwired: 1 in]
        n120 = call "Convert Milliseconds to Time.vi"("milliseconds"=w164) -> ("elapsed time"=w146:string)  [unwired: 1 in]
        n121 = Equal?(x=T4."Import .avi File", y=w135) -> (x = y?=w136:bool)
        n122 = Select(t=Interface_states."Watch" ("Enum"), s=w136, f=w133) -> (s? t:f=w132:T14)
        n123 = property on="Time in inner circle" class="Str"("Value"=w146) -> ()  [unwired: 2 in, 2 out]
        n124 = property on="Time in exterior circle" class="Str"("Value"=w148) -> ()  [unwired: 2 in, 2 out]
        n125 = property on="Time in middle circle" class="Str"("Value"=w147) -> ()  [unwired: 2 in, 2 out]
        n126 = property on="Time outside circles" class="Str"("Value"=w149) -> ()  [unwired: 2 in, 2 out]
      }
      frame "Watch" {
        n127 = Index Array(array=w206, index #1=0 ("index"), index #2=1 ("index")) -> (element #1=w184:refnum<class "Waveform data.lvclass">, element #2=w185:refnum<class "Waveform data.lvclass">)
        n128 = Equal?(x=w194, y=T16."Load video") -> (x = y?=w196:bool)
        n129 = case shown="False" w196 {
          tunnel: [w257 Interface_states."Watch" ("Enum")] -> w209
          tunnel: w208 -> [w279 _]
          tunnel: w185 -> [w220 w436]
          tunnel: [w278 w407] -> w205
          tunnel: [w239 w392] -> w204
          tunnel: [w276 T16."Idle" ("States")] -> w203
          tunnel: "Slide" -> [w277 w406]
          tunnel: [w244 _] -> w201
          tunnel: [w242 _] -> w200
          tunnel: [w246 w405] -> w199
          tunnel: [w245 w404] -> w198
          tunnel: [w240 _] -> w197
          tunnel: w194 -> [w265 _]
          tunnel: [w218 w397] -> w188
          tunnel: [w213 w396] -> w187
          tunnel: [w263 w422] -> w193
          tunnel: [w236 w393] -> w192
          tunnel: [w237 w395] -> w191
          tunnel: w190 -> [w258 _]
          tunnel: w189 -> [w238 _]
          frame False {
            w212 = u32 2 ("y")
            n130 = property on="file path" class="Path"() -> ("Value"=w224:path)  [unwired: 2 in, 2 out]
            n131 = Equal?(x=w224, y=path "") -> (x = y?=w222:bool)
            n132 = case shown="False" w222 {
              tunnel: [T16."Load video" ("Enum") T16."Idle" ("Enum")] -> w221
              frame False {
              }
              frame True {
              }
            }
            n133 = Select(t=T16."Play" ("Enum"), s="Play/Stop", f=w265) -> (s? t:f=w270:T16)
            n134 = Select(t=w221, s="Load file", f=w270) -> (s? t:f=w269:T16)
            n135 = Select(t=T16."Forward" ("Enum"), s="Forward", f=w269) -> (s? t:f=w268:T16)
            n136 = Select(t=T16."Rewind" ("Enum"), s="Rewind", f=w268) -> (s? t:f=w234:T16)
            n137 = control-ref of="Slide"() -> (w281:refnum<vi>)
            n138 = case shown="False" "Load file" {
              tunnel: [w390 _] -> w284
              tunnel: w281 -> [w389 _]
              tunnel: w279 -> [w388 _]
              tunnel: [w387 _] -> w239
              tunnel: [w386 w391] -> w276
              tunnel: w234 -> [w378 w391]
              tunnel: [w385 _] -> w235
              tunnel: "Play/Stop" -> [w384 _]
              tunnel: [w383 _] -> w218
              tunnel: [w382 _] -> w213
              tunnel: [w381 _] -> w263
              tunnel: [w380 _] -> w236
              tunnel: [w379 _] -> w237
              frame False {
                n139 = call-dynamic "Video feed info class VI - states.vi"("Video feed info in"=w388, "States"=w378, "Start/Stop"=w384, "Slide Refnum"=w389) -> ("Image"=w385:T5, "State output"=w386:T16, "Image Type"=w380:T3, "Current Frame"=w390:u32, "Video feed info out"=w387:refnum<class "Video feed info.lvclass">, "FPS"=w379:u32, "width"=w383:u32, "height"=w382:u32, "Number of Frames"=w381:u32)  [unwired: 4 in, 3 out]
              }
              frame True {
              }
            }
            n140 = Equal?(x=w234, y=T16."Play") -> (x = y?=w233:bool)
            n141 = Equal?(x=w234, y=T16."Rewind") -> (x = y?=w232:bool)
            n142 = Equal?(x=w234, y=T16."Forward") -> (x = y?=w231:bool)
            n143 = Compound Arithmetic op=OR(w233, w232, w231) -> (w230:bool)
            n144 = Divide(x=w218, y=w212) -> (x/y=w217:dbl)
            n145 = Divide(x=w213, y=w212) -> (x/y=w216:dbl)
            n146 = To Long Integer(number=w217) -> (32bit integer=w214:i32)
            n147 = To Long Integer(number=w216) -> (32bit integer=w215:i32)
            n148 = case shown="True" w230 {
              tunnel: [w287 w294] -> w240
              tunnel: w235 -> [w287 w309]
              tunnel: w214 -> [_ w290]
              tunnel: w215 -> [_ w291]
              frame False {
              }
              frame True {
                w298 = u32 0 items=["Frame", "Fill"] ("Drawing Mode (Frame)")
                w306 = u32 1 items=["Frame", "Fill"] ("Drawing Mode (Frame)")
                n149 = call "IMAQ Clear Overlay"("Image"=w309) -> ("Image Out"=w297:T5)  [unwired: 9 in, 1 out]
                n150 = stacked-sequence {
                  seq-local: [w315 _ _] -> [_ w326 _]
                  seq-local: [w314 _ _] -> [_ w328 _]
                  seq-local: [_ w320 _] -> [_ _ w376]
                  tunnel: [_ _ w375] -> w296
                  tunnel: w297 -> [w310 _ _]
                  frame #0 {
                    w314 = T3 0 items=["Grayscale (U8)", "Grayscale (I16)", "Grayscale (SGL)", "Complex (CSG)", "RGB (U32)", "HSL (U32)", "RGB (U64)", "Grayscale (U16)"] ("Image Type")
                    n151 = property on="Keep/Replace - video player" class="Bool (strict)"() -> ("Value"=w311:bool)  [unwired: 2 in, 2 out]
                    n152 = call "IMAQ Create"("Image Name"="image", "Image Type"=w314) -> ("New Image"=w316:T5)  [unwired: 3 in, 1 out]
                    n153 = property on="Range - video player" class="Clust (strict)"() -> ("Value"=w313:cluster{"Lower value":sgl, "Upper value":sgl})  [unwired: 2 in, 2 out]
                    n154 = property on="Replace Value - video player" class="DigNum (strict)"() -> ("Value"=w312:sgl)  [unwired: 2 in, 2 out]
                    n155 = call "IMAQ Cast Image"("Image Type"=w314, "Image Dst"=w316, "Image Src"=w310) -> ("Image Dst Out"=w317:T5)  [unwired: 7 in, 1 out]
                    n156 = call "IMAQ Threshold"("Replace Value"=w312, "Keep/Replace Value (Replace)"=w311, "Range"=w313, "Image Dst"=w316, "Image Src"=w317) -> ("Image Dst Out"=w315:T5)  [unwired: 5 in, 1 out]
                  }
                  frame #1 {
                    n157 = property on="Toggle Controls - video player" class="Clust (strict)"() -> ("Value"=w319:T7)  [unwired: 2 in, 2 out]
                    n158 = Unbundle(w319) -> ("Remove Border"=w325:bool, "Fill Hole"=w323:bool, "Remove Particles"=w322:bool, "Particle Filter"=w321:bool)
                    n159 = call "IMAQ Create"("Image Name"="morphology", "Image Type"=w328) -> ("New Image"=w324:T5)  [unwired: 3 in, 1 out]
                    n160 = stacked-sequence {
                      seq-local: [w329 _ _ _] -> [_ _ _ _]
                      seq-local: [_ w340 _ _] -> [_ _ _ _]
                      seq-local: [_ _ w350 _] -> [_ _ _ _]
                      tunnel: w326 -> [w332 w341 w351 w362]
                      tunnel: w325 -> [w331 _ _ _]
                      tunnel: w324 -> [w330 _ _ _]
                      tunnel: w323 -> [_ w342 _ _]
                      tunnel: [_ _ _ w361] -> w320
                      tunnel: w322 -> [_ _ w349 _]
                      tunnel: w321 -> [_ _ _ w360]
                      frame #0 {
                        n161 = case shown="True" w331 {
                          tunnel: w332 -> [w334 w339]
                          tunnel: w330 -> [_ w338]
                          tunnel: [w334 w337] -> w329
                          frame False {
                            n162 = property on="Connectivity 4/8: 4" class="Bool (strict)"("DisabledEnum"=T18."Disabled and Grayed Out" ("Disabled")) -> ()  [unwired: 2 in, 2 out]
                          }
                          frame True {
                            n163 = property on="Connectivity 4/8: 4" class="Bool (strict)"() -> ("Value"=w336:bool)  [unwired: 2 in, 2 out]
                            n164 = property on="Connectivity 4/8: 4" class="Bool (strict)"("DisabledEnum"=T18."Enabled" ("Disabled")) -> ()  [unwired: 2 in, 2 out]
                            n165 = call "IMAQ RejectBorder"("Image Dst"=w338, "Image Src"=w339, "Connectivity 4/8 (8)"=w336) -> ("Image Dst Out"=w337:T5)  [unwired: 3 in, 1 out]
                          }
                        }
                      }
                      frame #1 {
                        n166 = case shown="True" w342 {
                          tunnel: [w344 w348] -> w340
                          tunnel: w341 -> [w344 w347]
                          frame False {
                            n167 = property on="Connectivity 4/8: 5" class="Bool (strict)"("DisabledEnum"=T18."Disabled and Grayed Out" ("Disabled")) -> ()  [unwired: 2 in, 2 out]
                          }
                          frame True {
                            n168 = property on="Connectivity 4/8: 5" class="Bool (strict)"() -> ("Value"=w346:bool)  [unwired: 2 in, 2 out]
                            n169 = call "IMAQ FillHole"("Image Src"=w347, "Connectivity 4/8 (8)"=w346) -> ("Image Dst Out"=w348:T5)  [unwired: 4 in, 1 out]
                            n170 = property on="Connectivity 4/8: 5" class="Bool (strict)"("DisabledEnum"=T18."Enabled" ("Disabled")) -> ()  [unwired: 2 in, 2 out]
                          }
                        }
                      }
                      frame #2 {
                        n171 = case shown="True" w349 {
                          tunnel: w351 -> [w353 w359]
                          tunnel: [w353 w358] -> w350
                          frame False {
                            w352 = T18."Disabled and Grayed Out" ("Disabled")
                            n172 = property on="Low Pass/High Pass: video player" class="Bool (strict)"("DisabledEnum"=w352) -> ()  [unwired: 2 in, 2 out]
                            n173 = property on="Square/Hexagon: video player" class="Bool (strict)"("DisabledEnum"=w352) -> ()  [unwired: 2 in, 2 out]
                            n174 = property on="Number of Erosion: video player" class="DigNum (strict)"("DisabledEnum"=w352) -> ()  [unwired: 2 in, 2 out]
                          }
                          frame True {
                            w357 = T18."Enabled" ("Disabled")
                            n175 = property on="Square/Hexagon: video player" class="Bool (strict)"() -> ("Value"=w356:bool)  [unwired: 2 in, 2 out]
                            n176 = property on="Number of Erosion: video player" class="DigNum (strict)"() -> ("Value"=w355:i32)  [unwired: 2 in, 2 out]
                            n177 = property on="Low Pass/High Pass: video player" class="Bool (strict)"() -> ("Value"=w354:bool)  [unwired: 2 in, 2 out]
                            n178 = call "IMAQ RemoveParticle"("Connectivity 4/8 (8)"=w356, "Low Pass/High Pass (Low)"=w354, "Number of Erosion"=w355, "Image Src"=w359) -> ("Image Dst Out"=w358:T5)  [unwired: 6 in, 1 out]
                            n179 = property on="Low Pass/High Pass: video player" class="Bool (strict)"("DisabledEnum"=w357) -> ()  [unwired: 2 in, 2 out]
                            n180 = property on="Square/Hexagon: video player" class="Bool (strict)"("DisabledEnum"=w357) -> ()  [unwired: 2 in, 2 out]
                            n181 = property on="Number of Erosion: video player" class="DigNum (strict)"("DisabledEnum"=w357) -> ()  [unwired: 2 in, 2 out]
                          }
                        }
                      }
                      frame #3 {
                        n182 = case shown="True" w360 {
                          tunnel: w362 -> [w364 w372]
                          tunnel: [w364 w371] -> w361
                          frame False {
                            w363 = T18."Disabled and Grayed Out" ("Disabled")
                            n183 = property on="ROI Descriptor - video player" class="Clust (strict)"("DisabledEnum"=w363) -> ()  [unwired: 2 in, 2 out]
                            n184 = property on="Keep/Remove Particles - video player" class="Bool (strict)"("DisabledEnum"=w363) -> ()  [unwired: 2 in, 2 out]
                            n185 = property on="Connectivity 4/8: 6" class="Bool (strict)"("DisabledEnum"=w363) -> ()  [unwired: 2 in, 2 out]
                            n186 = property on="Selection Values - video player" class="Arr (strict)"("DisabledEnum"=w363) -> ()  [unwired: 2 in, 2 out]
                          }
                          frame True {
                            w369 = T18."Enabled" ("Disabled")
                            n187 = property on="Selection Values - video player" class="Arr (strict)"() -> ("Value"=w366:T10)  [unwired: 2 in, 2 out]
                            n188 = property on="Keep/Remove Particles - video player" class="Bool (strict)"() -> ("Value"=w365:bool)  [unwired: 2 in, 2 out]
                            n189 = property on="Connectivity 4/8: 6" class="Bool (strict)"() -> ("Value"=w367:bool)  [unwired: 2 in, 2 out]
                            n190 = property on="ROI Descriptor - video player" class="Clust (strict)"() -> ("Value"=w368:T15)  [unwired: 2 in, 2 out]
                            n191 = call "IMAQ Particle Filter 3"("Image Src"=w372, "Connectivity 4/8 (8)"=w367, "ROI Descriptor"=w368, "Selection Values"=w366, "Keep/Remove Particles (F)"=w365, "Fill Holes? (F)"=TRUE) -> ("Image Dst Out"=w371:T5)  [unwired: 7 in, 2 out]
                            n192 = property on="Connectivity 4/8: 6" class="Bool (strict)"("DisabledEnum"=w369) -> ()  [unwired: 2 in, 2 out]
                            n193 = property on="Keep/Remove Particles - video player" class="Bool (strict)"("DisabledEnum"=w369) -> ()  [unwired: 2 in, 2 out]
                            n194 = property on="Selection Values - video player" class="Arr (strict)"("DisabledEnum"=w369) -> ()  [unwired: 2 in, 2 out]
                            n195 = property on="ROI Descriptor - video player" class="Clust (strict)"("DisabledEnum"=w369) -> ()  [unwired: 2 in, 2 out]
                          }
                        }
                      }
                    }
                  }
                  frame #2 {
                    n196 = property on="Min Radius - video player" class="DigNum (strict)"() -> ("Value"=w374:sgl)  [unwired: 2 in, 2 out]
                    n197 = property on="Max Radius - video player" class="DigNum (strict)"() -> ("Value"=w373:sgl)  [unwired: 2 in, 2 out]
                    n198 = call "IMAQ Find Circles"("Max Radius"=w373, "Min Radius"=w374, "Image Src"=w376) -> ("Circles Data"=w377:T11)  [unwired: 5 in, 3 out]
                    n199 = call "sort circles.vi"("circles"=w377) -> ("Sorted circles"=w375:T11)
                  }
                }
                n200 = call "Extract Circle Information.vi"("Circle Data"=w296) -> ("Circle bounding rectangle"=w307:cluster{i32, i32, i32, i32}, "Circle x and y"=w295:cluster{"Pos. X":i32, "Pos. Y":i32})
                n201 = Bundle By Name(cluster=w295, "Pos. X"=w290, "Pos. Y"=w291) -> (w302:cluster{"Pos. X":i32, "Pos. Y":i32})
                n202 = call "Create bounding rectangle based on center.vi"("x center"=w290, "y center"=w291, "distance from x/y center"=i16 3) -> ("bounding rectangle coordinates"=w288:cluster{i16, i16, i16, i16})
                n203 = property on="center color" class="ColBox"() -> ("Value"=w303:u32)  [unwired: 2 in, 2 out]
                n204 = call "calculate angles.vi"("Midpoint x and y"=w302, "point"=w295) -> ("angle (degrees)"=w300:dbl)
                n205 = call "Find Distance Between Points.vi"("position 2"=w302, "position 1"=w295) -> ()  [unwired: 1 out]
                n206 = call "IMAQ Overlay Oval"("Color"=w303, "Drawing Mode (Frame)"=w306, "Bounding Rectangle"=w288, "Image"=w297) -> ("Image Out"=w301:T5)  [unwired: 6 in, 1 out]
                n207 = call "Create bounding rectangle based on center.vi"("x center"=w290, "y center"=w291, "distance from x/y center"=i16 5) -> ("bounding rectangle coordinates"=w289:cluster{i16, i16, i16, i16})
                n208 = call "IMAQ Overlay Arc"("End Angle (degrees)"=w300, "Color"=w303, "Start Angle (degrees)"=0.0, "Drawing Mode (Frame)"=w298, "Bounding Rectangle"=w289, "Image"=w301) -> ("Image Out"=w308:T5)  [unwired: 4 in, 1 out]
                n209 = call "IMAQ Overlay Line"("Color"=w303, "End Point"=w295, "Start Point"=w302, "Image"=w308) -> ("Image Out"=w304:T5)  [unwired: 6 in, 1 out]
                n210 = property on="dot color" class="ColBox"() -> ("Value"=w305:u32)  [unwired: 2 in, 2 out]
                n211 = call "IMAQ Overlay Oval"("Color"=w305, "Drawing Mode (Frame)"=w306, "Bounding Rectangle"=w307, "Image"=w304) -> ("Image Out"=w294:T5)  [unwired: 6 in, 1 out]
              }
            }
            n212 = Unbundle(w277) -> (w280:u32, w250:u32, w249:u32)
            n213 = property on="Tab Control" class="TabCtl (strict)"() -> ("Value"=w219:T4)  [unwired: 2 in, 2 out]
            n214 = call-dynamic "Waveform data class VI - retrieve waveform data.vi"("Waveform data in"=w220) -> ("Waveform data out"=w278:refnum<class "Waveform data.lvclass">, "angles"=w283:dbl[], "displacement"=w282:dbl[])  [unwired: 11 in, 1 out]
            n215 = Subtract(x=w280, y=w250) -> (x-y=w226:u32)
            n216 = Subtract(x=w249, y=w250) -> (x-y=w247:u32)
            n217 = Not Equal?(x=w219, y=T4."Import .avi File") -> (x != y?=w262:bool)
            n218 = To Long Integer(number=w226) -> (32bit integer=w251:i32)
            n219 = Index Array(array=w283, index=w284) -> (element=w246:dbl)
            n220 = Index Array(array=w282, index=w284) -> (element=w245:dbl)
            n221 = Array Subset(array=w283, index=w250, length=w226) -> (w275:dbl[])
            n222 = Array Subset(array=w282, index=w250, length=w226) -> (w274:dbl[])
            n223 = Select(t=Interface_states."Idle" ("Enum"), s=w262, f=Interface_states."Watch") -> (s? t:f=w260:T14)
            n224 = Initialize Array(-200 ("element"), w251) -> (w248:i32[])
            n225 = Initialize Array(100 ("element"), w226) -> ()  [unwired: 1 out]
            n226 = Replace Array Subset(array=w248, new element=w246, index=w247) -> (w243:i32[])
            n227 = Replace Array Subset(array=w248, new element=w245, index=w247) -> (w241:i32[])
            n228 = Select(t=Interface_states."Analyze", s=w258, f=w260) -> (s? t:f=w259:T14)
            n229 = Build Array(w275, w243) -> (w244:dbl[][])
            n230 = Build Array(w274, w241) -> (w242:dbl[][])
            n231 = Select(t=Interface_states."Reset", s=w238, f=w259) -> (s? t:f=w257:T14)
          }
          frame True {
            w402 = u8 0 ("Plot.Line Style")
            w403 = u8 2 ("Plot.Point Style")
            w401 = u8 0 ("Plot.Plot Interpolation")
            w400 = u8 5 ("Plot.Line Width")
            w399 = u32 1 ("Active Plot")
            n232 = control-ref of="Slide"() -> (w427:refnum<vi>)
            n233 = call-dynamic "Video feed info class VI - states.vi"("Video feed info in"=refnum<class "Video feed info.lvclass"> refnum ("Video feed info.lvclass"), "States"=T16."Load video" ("Enum"), "start path"="file path", "Slide Refnum"=w427) -> ("file path"=w394:path, "Image Type"=w393:T3, "Video feed info out"=w431:refnum<class "Video feed info.lvclass">, "FPS"=w395:u32, "width"=w397:u32, "height"=w396:u32, "Number of Frames"=w422:u32)  [unwired: 4 in, 5 out]
            n234 = To Long Integer(number=w422) -> (32bit integer=w432:i32)
            n235 = property on="file path" class="Path"("Value"=w394) -> ()  [unwired: 2 in, 2 out]
            n236 = call-dynamic "Video feed info class VI - states.vi"("Video feed info in"=w431, "States"=T16."Idle", "Slide Refnum"=w427) -> ("Video feed info out"=w430:refnum<class "Video feed info.lvclass">)  [unwired: 5 in, 11 out]
            n237 = for {
              N: w432 -> [_]
              shift-right: [w467] -> w392
              shift-left: w430 -> [w475]
              shift-right: [w464] -> w407
              shift-left: w436 -> [w465]
              i -> [w471]
              w446 = u32 2 ("y")
              w449 = u32 0 items=["Frame", "Fill"] ("Drawing Mode (Frame)")
              w459 = u32 1 items=["Frame", "Fill"] ("Drawing Mode (Frame)")
              w470 = 0
              n238 = control-ref of="Slide"() -> (w466:refnum<vi>)
              n239 = Bundle(w471, w470, w470) -> (w469:cluster{i32, i32, i32})  [unwired: 1 in]
              n240 = property on="Slide" class="Slide (strict)"("Value"=w469) -> ()  [unwired: 2 in, 2 out]
              n241 = call-dynamic "Video feed info class VI - states.vi"("Video feed info in"=w475, "States"=T16."Play", "Start/Stop"=FALSE, "Slide Refnum"=w466) -> ("Image"=w473:T5, "Video feed info out"=w467:refnum<class "Video feed info.lvclass">, "width"=w445:u32, "height"=w444:u32)  [unwired: 4 in, 8 out]
              n242 = call "IMAQ Clear Overlay"("Image"=w473) -> ("Image Out"=w453:T5)  [unwired: 9 in, 1 out]
              n243 = stacked-sequence {
                seq-local: [w477 _ _] -> [_ w491 _]
                seq-local: [w476 _ _] -> [_ w494 _]
                seq-local: [_ w485 _] -> [_ _ w540]
                tunnel: w453 -> [w478 _ _]
                tunnel: [_ _ w539] -> w472
                frame #0 {
                  w476 = T3 0 items=["Grayscale (U8)", "Grayscale (I16)", "Grayscale (SGL)", "Complex (CSG)", "RGB (U32)", "HSL (U32)", "RGB (U64)", "Grayscale (U16)"] ("Image Type")
                  n244 = call "IMAQ Create"("Image Name"="image", "Image Type"=w476) -> ("New Image"=w479:T5)  [unwired: 3 in, 1 out]
                  n245 = call "IMAQ Cast Image"("Image Type"=w476, "Image Dst"=w479, "Image Src"=w478) -> ("Image Dst Out"=w483:T5)  [unwired: 7 in, 1 out]
                  n246 = call "IMAQ Threshold"("Replace Value"="Replace Value - video player", "Keep/Replace Value (Replace)"="Keep/Replace - video player", "Range"="Range - video player", "Image Dst"=w479, "Image Src"=w483) -> ("Image Dst Out"=w477:T5)  [unwired: 5 in, 1 out]
                }
                frame #1 {
                  n247 = Unbundle("Toggle Controls - video player") -> ("Remove Border"=w490:bool, "Fill Hole"=w488:bool, "Remove Particles"=w487:bool, "Particle Filter"=w486:bool)
                  n248 = call "IMAQ Create"("Image Name"="morphology", "Image Type"=w494) -> ("New Image"=w489:T5)  [unwired: 3 in, 1 out]
                  n249 = stacked-sequence {
                    seq-local: [w495 _ _ _] -> [_ _ _ _]
                    seq-local: [_ w506 _ _] -> [_ _ _ _]
                    seq-local: [_ _ w516 _] -> [_ _ _ _]
                    tunnel: w491 -> [w498 w507 w517 w528]
                    tunnel: w490 -> [w497 _ _ _]
                    tunnel: w489 -> [w496 _ _ _]
                    tunnel: w488 -> [_ w508 _ _]
                    tunnel: [_ _ _ w527] -> w485
                    tunnel: w487 -> [_ _ w515 _]
                    tunnel: w486 -> [_ _ _ w526]
                    frame #0 {
                      n250 = case shown="True" w497 {
                        tunnel: w498 -> [w500 w504]
                        tunnel: w496 -> [_ w503]
                        tunnel: [w500 w502] -> w495
                        frame False {
                          n251 = property on="Connectivity 4/8: 4" class="Bool (strict)"("DisabledEnum"=T18."Disabled and Grayed Out" ("Disabled")) -> ()  [unwired: 2 in, 2 out]
                        }
                        frame True {
                          n252 = property on="Connectivity 4/8: 4" class="Bool (strict)"("DisabledEnum"=T18."Enabled" ("Disabled")) -> ()  [unwired: 2 in, 2 out]
                          n253 = call "IMAQ RejectBorder"("Image Dst"=w503, "Image Src"=w504, "Connectivity 4/8 (8)"="Connectivity 4/8: 4") -> ("Image Dst Out"=w502:T5)  [unwired: 3 in, 1 out]
                        }
                      }
                    }
                    frame #1 {
                      n254 = case shown="True" w508 {
                        tunnel: [w510 w514] -> w506
                        tunnel: w507 -> [w510 w512]
                        frame False {
                          n255 = property on="Connectivity 4/8: 5" class="Bool (strict)"("DisabledEnum"=T18."Disabled and Grayed Out" ("Disabled")) -> ()  [unwired: 2 in, 2 out]
                        }
                        frame True {
                          n256 = call "IMAQ FillHole"("Image Src"=w512, "Connectivity 4/8 (8)"="Connectivity 4/8: 5") -> ("Image Dst Out"=w514:T5)  [unwired: 4 in, 1 out]
                          n257 = property on="Connectivity 4/8: 5" class="Bool (strict)"("DisabledEnum"=T18."Enabled" ("Disabled")) -> ()  [unwired: 2 in, 2 out]
                        }
                      }
                    }
                    frame #2 {
                      n258 = case shown="True" w515 {
                        tunnel: w517 -> [w518 w521]
                        tunnel: [w518 w520] -> w516
                        frame False {
                          w519 = T18."Disabled and Grayed Out" ("Disabled")
                          n259 = property on="Low Pass/High Pass: video player" class="Bool (strict)"("DisabledEnum"=w519) -> ()  [unwired: 2 in, 2 out]
                          n260 = property on="Square/Hexagon: video player" class="Bool (strict)"("DisabledEnum"=w519) -> ()  [unwired: 2 in, 2 out]
                          n261 = property on="Number of Erosion: video player" class="DigNum (strict)"("DisabledEnum"=w519) -> ()  [unwired: 2 in, 2 out]
                        }
                        frame True {
                          w522 = T18."Enabled" ("Disabled")
                          n262 = call "IMAQ RemoveParticle"("Connectivity 4/8 (8)"="Square/Hexagon: video player", "Low Pass/High Pass (Low)"="Low Pass/High Pass: video player", "Number of Erosion"="Number of Erosion: video player", "Image Src"=w521) -> ("Image Dst Out"=w520:T5)  [unwired: 6 in, 1 out]
                          n263 = property on="Low Pass/High Pass: video player" class="Bool (strict)"("DisabledEnum"=w522) -> ()  [unwired: 2 in, 2 out]
                          n264 = property on="Square/Hexagon: video player" class="Bool (strict)"("DisabledEnum"=w522) -> ()  [unwired: 2 in, 2 out]
                          n265 = property on="Number of Erosion: video player" class="DigNum (strict)"("DisabledEnum"=w522) -> ()  [unwired: 2 in, 2 out]
                        }
                      }
                    }
                    frame #3 {
                      n266 = case shown="True" w526 {
                        tunnel: w528 -> [w530 w538]
                        tunnel: [w530 w537] -> w527
                        frame False {
                          w529 = T18."Disabled and Grayed Out" ("Disabled")
                          n267 = property on="ROI Descriptor - video player" class="Clust (strict)"("DisabledEnum"=w529) -> ()  [unwired: 2 in, 2 out]
                          n268 = property on="Keep/Remove Particles - video player" class="Bool (strict)"("DisabledEnum"=w529) -> ()  [unwired: 2 in, 2 out]
                          n269 = property on="Connectivity 4/8: 6" class="Bool (strict)"("DisabledEnum"=w529) -> ()  [unwired: 2 in, 2 out]
                          n270 = property on="Selection Values - video player" class="Arr (strict)"("DisabledEnum"=w529) -> ()  [unwired: 2 in, 2 out]
                        }
                        frame True {
                          w531 = T18."Enabled" ("Disabled")
                          n271 = call "IMAQ Particle Filter 3"("Image Src"=w538, "Connectivity 4/8 (8)"="Connectivity 4/8: 6", "ROI Descriptor"="ROI Descriptor - video player", "Selection Values"="Selection Values - video player", "Keep/Remove Particles (F)"="Keep/Remove Particles - video player", "Fill Holes? (F)"=TRUE) -> ("Image Dst Out"=w537:T5)  [unwired: 7 in, 2 out]
                          n272 = property on="Connectivity 4/8: 6" class="Bool (strict)"("DisabledEnum"=w531) -> ()  [unwired: 2 in, 2 out]
                          n273 = property on="Keep/Remove Particles - video player" class="Bool (strict)"("DisabledEnum"=w531) -> ()  [unwired: 2 in, 2 out]
                          n274 = property on="Selection Values - video player" class="Arr (strict)"("DisabledEnum"=w531) -> ()  [unwired: 2 in, 2 out]
                          n275 = property on="ROI Descriptor - video player" class="Clust (strict)"("DisabledEnum"=w531) -> ()  [unwired: 2 in, 2 out]
                        }
                      }
                    }
                  }
                }
                frame #2 {
                  n276 = call "IMAQ Find Circles"("Max Radius"="Max Radius - video player", "Min Radius"="Min Radius - video player", "Image Src"=w540) -> ("Circles Data"=w541:T11)  [unwired: 5 in, 3 out]
                  n277 = call "sort circles.vi"("circles"=w541) -> ("Sorted circles"=w539:T11)
                }
              }
              n278 = Divide(x=w445, y=w446) -> (x/y=w448:dbl)
              n279 = Divide(x=w444, y=w446) -> (x/y=w447:dbl)
              n280 = To Long Integer(number=w448) -> (32bit integer=w439:i32)
              n281 = To Long Integer(number=w447) -> (32bit integer=w440:i32)
              n282 = call "Extract Circle Information.vi"("Circle Data"=w472) -> ("Circle bounding rectangle"=w460:cluster{i32, i32, i32, i32}, "Circle x and y"=w454:cluster{"Pos. X":i32, "Pos. Y":i32})
              n283 = Bundle By Name(cluster=w454, "Pos. X"=w439, "Pos. Y"=w440) -> (w455:cluster{"Pos. X":i32, "Pos. Y":i32})
              n284 = property on="center color" class="ColBox"() -> ("Value"=w456:u32)  [unwired: 2 in, 2 out]
              n285 = call "Create bounding rectangle based on center.vi"("x center"=w439, "y center"=w440, "distance from x/y center"=i16 3) -> ("bounding rectangle coordinates"=w443:cluster{i16, i16, i16, i16})
              n286 = call "calculate angles.vi"("Midpoint x and y"=w455, "point"=w454) -> ("angle (degrees)"=w451:dbl)
              n287 = call "Find Distance Between Points.vi"("position 2"=w455, "position 1"=w454) -> ("distance"=w463:dbl)
              n288 = call "IMAQ Overlay Oval"("Color"=w456, "Drawing Mode (Frame)"=w459, "Bounding Rectangle"=w443, "Image"=w453) -> ("Image Out"=w452:T5)  [unwired: 6 in, 1 out]
              n289 = call "Create bounding rectangle based on center.vi"("x center"=w439, "y center"=w440, "distance from x/y center"=i16 5) -> ("bounding rectangle coordinates"=w438:cluster{i16, i16, i16, i16})
              n290 = call "IMAQ Overlay Arc"("End Angle (degrees)"=w451, "Color"=w456, "Start Angle (degrees)"=0.0, "Drawing Mode (Frame)"=w449, "Bounding Rectangle"=w438, "Image"=w452) -> ("Image Out"=w462:T5)  [unwired: 4 in, 1 out]
              n291 = call "IMAQ Overlay Line"("Color"=w456, "End Point"=w454, "Start Point"=w455, "Image"=w462) -> ("Image Out"=w457:T5)  [unwired: 6 in, 1 out]
              n292 = property on="dot color" class="ColBox"() -> ("Value"=w458:u32)  [unwired: 2 in, 2 out]
              n293 = call "IMAQ Overlay Oval"("Color"=w458, "Drawing Mode (Frame)"=w459, "Bounding Rectangle"=w460, "Image"=w457) -> ("Image Out"=w461:T5)  [unwired: 6 in, 1 out]
              n294 = call-dynamic "Waveform data class VI - add waveform data.vi"("Waveform data in"=w465, "angle"=w451, "displacement"=w463) -> ("Waveform data out"=w464:refnum<class "Waveform data.lvclass">)  [unwired: 11 in, 1 out]
              n295 = property on="Image" class="ImageControl"("Value"=w461) -> ()  [unwired: 2 in, 2 out]
            }
            n296 = property on="displacement - vp" class="WFGraph (strict)"("YScale.Maximum"=w397, "YScale.Minimum"=0.0 ("Y Scale.Range:Minimum")) -> ()  [unwired: 2 in, 2 out]
            n297 = call-dynamic "Video feed info class VI - retrieve beginning-end cursor states.vi"("Video feed info in"=w392) -> ("Higher Cursor value"=w424:u32, "Lower Cursor value"=w425:u32)  [unwired: 7 in, 2 out]
            n298 = Unbundle(w406) -> (w419:u32, w413:u32, w412:u32)
            n299 = Bundle("Higher Cursor value"=w424, "Lower Cursor value"=w425, "Higher Cursor value"=u32 0) -> (w428:T20)  [unwired: 1 in]
            n300 = call-dynamic "Waveform data class VI - retrieve waveform data.vi"("Waveform data in"=w407) -> ("angles"=w421:dbl[], "displacement"=w420:dbl[])  [unwired: 11 in, 2 out]
            n301 = Subtract(x=w412, y=w413) -> (x-y=w410:u32)
            n302 = property on="Slide" class="Slide (strict)"("Value"=w428) -> ()  [unwired: 2 in, 2 out]
            n303 = Subtract(x=w419, y=w413) -> (x-y=w416:u32)
            n304 = Index Array(array=w421) -> (element=w405:dbl)  [unwired: 1 in]
            n305 = Index Array(array=w420) -> (element=w404:dbl)  [unwired: 1 in]
            n306 = To Long Integer(number=w416) -> (32bit integer=w414:i32)
            n307 = Array Subset(array=w421, index=w413, length=w416) -> (w418:dbl[])
            n308 = Array Subset(array=w420, index=w413, length=w416) -> (w417:dbl[])
            n309 = Initialize Array(0 ("element"), w414) -> (w411:i32[])
            n310 = Replace Array Subset(array=w411, new element=w405, index=w410) -> (w409:i32[])
            n311 = Replace Array Subset(array=w411, new element=w404, index=w410) -> (w408:i32[])
            n312 = Build Array(w417, w408) -> ()  [unwired: 1 out]
            n313 = Build Array(w418, w409) -> ()  [unwired: 1 out]
            n314 = property on="angles - vp" class="WFGraph (strict)"("Active Plot"=w399, "Plot.Line Width"=w400, "Plot.Plot Interpolation"=w401, "Plot.Line Style"=w402, "Plot.Point Style"=w403) -> ()  [unwired: 2 in, 2 out]
            n315 = property on="displacement - vp" class="WFGraph (strict)"("Active Plot"=w399, "Plot.Line Width"=w400, "Plot.Plot Interpolation"=w401, "Plot.Line Style"=w402, "Plot.Point Style"=w403) -> ()  [unwired: 2 in, 2 out]
          }
        }
        "angles - vp" <- w201
        "displacement - vp" <- w200
        "angle (degrees) - vp" <- w199
        "displacement - vp" <- w198
        "FPS" <- w191
        "width" <- w188
        "height" <- w187
        "Number of Frames" <- w193
        "Image video" <- w192
        "Image" <- w197
        n316 = Build Array(w184, w205) -> (w183:refnum<class "Waveform data.lvclass">[])
      }
      frame "Record" {
        w576 = u32 1 items=["Horizontal", "Vertical", "Central", "1st Diagonal", "2nd Diagonal"] ("Type of Symmetry")
        w631 = i16 2 ("y")
        w602 = i16 2 ("radius")
        w640 = FALSE ("fill?(F)")
        w560 = TRUE ("fill?(F)")
        n317 = Index Array(array=w617, index #1=0 ("index"), index #2=1 ("index")) -> (element #1=w614:refnum<class "Waveform data.lvclass">, element #2=w613:refnum<class "Waveform data.lvclass">)
        n318 = Not(x=w662) -> (.not. x?=w661:bool)
        n319 = call "Camera acquisition.vi"("camera feed"="camera feed", "Stop (F)"=w661) -> ("Image Out"=w577:T5, "Image Number"=→"Image Number":u32, "Frame Rate"=w574:dbl, "Stopped"=w660:bool)  [unwired: 20 in, 2 out]
        "Frame Rate" <- w574
        n320 = Reciprocal(x=w574) -> (1/x=w573:dbl)
        n321 = property on="distance" class="WFChart (strict)"("XScale.Multiplier"=w573) -> ()  [unwired: 2 in, 2 out]
        n322 = property on="angles" class="WFChart (strict)"("XScale.Multiplier"=w573) -> ()  [unwired: 2 in, 2 out]
        n323 = call "IMAQ Symmetry"("Type of Symmetry"=w576, "Image Src"=w577) -> ("Image Dst Out"=w578:T5)  [unwired: 3 in, 1 out]
        n324 = stacked-sequence {
          seq-local: [w791 _ _] -> [_ w804 _]
          seq-local: ["Image Type" _ _] -> [_ w807 _]
          seq-local: [_ w798 _] -> [_ _ w853]
          tunnel: w578 -> [w787 _ _]
          tunnel: [_ _ w852] -> w664
          tunnel: [w789 _ _] -> w632
          tunnel: [w788 _ _] -> w633
          frame #0 {
            n325 = call "IMAQ GetImageInfo"("Image"=w787) -> ("Y Resolution"=w788:i32, "X Resolution"=w789:i32)  [unwired: 3 in, 6 out]
            "X Resolution" <- w789
            "Y Resolution" <- w788
            n326 = call "IMAQ Create"("Image Name"="image", "Image Type"="Image Type") -> ("New Image"=w792:T5)  [unwired: 3 in, 1 out]
            n327 = call "IMAQ Cast Image"("Image Type"="Image Type", "Image Dst"=w792, "Image Src"=w787) -> ("Image Dst Out"=w796:T5)  [unwired: 7 in, 1 out]
            n328 = call "IMAQ Threshold"("Replace Value"="Replace Value", "Keep/Replace Value (Replace)"="Keep/Replace", "Range"="Range", "Image Dst"=w792, "Image Src"=w796) -> ("Image Dst Out"=w791:T5)  [unwired: 5 in, 1 out]
            "raw display" <- w787
          }
          frame #1 {
            n329 = Unbundle("Toggle Controls") -> ("Remove Border"=w803:bool, "Fill Hole"=w801:bool, "Remove Particles"=w800:bool, "Particle Filter"=w799:bool)
            n330 = call "IMAQ Create"("Image Name"="morphology", "Image Type"=w807) -> ("New Image"=w802:T5)  [unwired: 3 in, 1 out]
            n331 = stacked-sequence {
              seq-local: [w808 _ _ _] -> [_ _ _ _]
              seq-local: [_ w819 _ _] -> [_ _ _ _]
              seq-local: [_ _ w829 _] -> [_ _ _ _]
              tunnel: w804 -> [w811 w820 w830 w841]
              tunnel: w803 -> [w810 _ _ _]
              tunnel: w802 -> [w809 _ _ _]
              tunnel: w801 -> [_ w821 _ _]
              tunnel: [_ _ _ w840] -> w798
              tunnel: w800 -> [_ _ w828 _]
              tunnel: w799 -> [_ _ _ w839]
              frame #0 {
                n332 = case shown="True" w810 {
                  tunnel: w811 -> [w813 w817]
                  tunnel: w809 -> [_ w816]
                  tunnel: [w813 w815] -> w808
                  frame False {
                    n333 = property on="Connectivity 4/8: 3" class="Bool (strict)"("DisabledEnum"=T18."Disabled and Grayed Out" ("Disabled")) -> ()  [unwired: 2 in, 2 out]
                  }
                  frame True {
                    n334 = property on="Connectivity 4/8: 3" class="Bool (strict)"("DisabledEnum"=T18."Enabled" ("Disabled")) -> ()  [unwired: 2 in, 2 out]
                    n335 = call "IMAQ RejectBorder"("Image Dst"=w816, "Image Src"=w817, "Connectivity 4/8 (8)"="Connectivity 4/8: 3") -> ("Image Dst Out"=w815:T5)  [unwired: 3 in, 1 out]
                  }
                }
              }
              frame #1 {
                n336 = case shown="True" w821 {
                  tunnel: [w823 w827] -> w819
                  tunnel: w820 -> [w823 w825]
                  frame False {
                    n337 = property on="Connectivity 4/8: 2" class="Bool (strict)"("DisabledEnum"=T18."Disabled and Grayed Out" ("Disabled")) -> ()  [unwired: 2 in, 2 out]
                  }
                  frame True {
                    n338 = call "IMAQ FillHole"("Image Src"=w825, "Connectivity 4/8 (8)"="Connectivity 4/8: 2") -> ("Image Dst Out"=w827:T5)  [unwired: 4 in, 1 out]
                    n339 = property on="Connectivity 4/8: 2" class="Bool (strict)"("DisabledEnum"=T18."Enabled" ("Disabled")) -> ()  [unwired: 2 in, 2 out]
                  }
                }
              }
              frame #2 {
                n340 = case shown="True" w828 {
                  tunnel: w830 -> [w831 w834]
                  tunnel: [w831 w833] -> w829
                  frame False {
                    w832 = T18."Disabled and Grayed Out" ("Disabled")
                    n341 = property on="Low Pass/High Pass:" class="Bool (strict)"("DisabledEnum"=w832) -> ()  [unwired: 2 in, 2 out]
                    n342 = property on="Square/Hexagon:" class="Bool (strict)"("DisabledEnum"=w832) -> ()  [unwired: 2 in, 2 out]
                    n343 = property on="Number of Erosion:" class="DigNum (strict)"("DisabledEnum"=w832) -> ()  [unwired: 2 in, 2 out]
                  }
                  frame True {
                    w835 = T18."Enabled" ("Disabled")
                    n344 = call "IMAQ RemoveParticle"("Connectivity 4/8 (8)"="Square/Hexagon:", "Low Pass/High Pass (Low)"="Low Pass/High Pass:", "Number of Erosion"="Number of Erosion:", "Image Src"=w834) -> ("Image Dst Out"=w833:T5)  [unwired: 6 in, 1 out]
                    n345 = property on="Low Pass/High Pass:" class="Bool (strict)"("DisabledEnum"=w835) -> ()  [unwired: 2 in, 2 out]
                    n346 = property on="Square/Hexagon:" class="Bool (strict)"("DisabledEnum"=w835) -> ()  [unwired: 2 in, 2 out]
                    n347 = property on="Number of Erosion:" class="DigNum (strict)"("DisabledEnum"=w835) -> ()  [unwired: 2 in, 2 out]
                  }
                }
              }
              frame #3 {
                n348 = case shown="True" w839 {
                  tunnel: w841 -> [w843 w851]
                  tunnel: [w843 w850] -> w840
                  frame False {
                    w842 = T18."Disabled and Grayed Out" ("Disabled")
                    n349 = property on="ROI Descriptor" class="Clust (strict)"("DisabledEnum"=w842) -> ()  [unwired: 2 in, 2 out]
                    n350 = property on="Keep/Remove Particles" class="Bool (strict)"("DisabledEnum"=w842) -> ()  [unwired: 2 in, 2 out]
                    n351 = property on="Connectivity 4/8:" class="Bool (strict)"("DisabledEnum"=w842) -> ()  [unwired: 2 in, 2 out]
                    n352 = property on="Selection Values" class="Arr (strict)"("DisabledEnum"=w842) -> ()  [unwired: 2 in, 2 out]
                  }
                  frame True {
                    w844 = T18."Enabled" ("Disabled")
                    n353 = call "IMAQ Particle Filter 3"("Image Src"=w851, "Connectivity 4/8 (8)"="Connectivity 4/8:", "ROI Descriptor"="ROI Descriptor", "Selection Values"="Selection Values", "Keep/Remove Particles (F)"="Keep/Remove Particles", "Fill Holes? (F)"=TRUE) -> ("Image Dst Out"=w850:T5)  [unwired: 7 in, 2 out]
                    n354 = property on="Connectivity 4/8:" class="Bool (strict)"("DisabledEnum"=w844) -> ()  [unwired: 2 in, 2 out]
                    n355 = property on="Keep/Remove Particles" class="Bool (strict)"("DisabledEnum"=w844) -> ()  [unwired: 2 in, 2 out]
                    n356 = property on="Selection Values" class="Arr (strict)"("DisabledEnum"=w844) -> ()  [unwired: 2 in, 2 out]
                    n357 = property on="ROI Descriptor" class="Clust (strict)"("DisabledEnum"=w844) -> ()  [unwired: 2 in, 2 out]
                  }
                }
              }
            }
            "Filtered Image" <- w798
          }
          frame #2 {
            n358 = call "IMAQ Find Circles"("Max Radius"="Max Radius", "Min Radius"="Min Radius", "Image Src"=w853) -> ("Circles Data"=w854:T11, "Image Dst Out"=→"Circles":T5)  [unwired: 5 in, 2 out]
            n359 = call "sort circles.vi"("circles"=w854) -> ("Sorted circles"=w852:T11)
            "Circles Data" <- w852
          }
        }
        n360 = To Word Integer(number=w633) -> (16bit integer=w590:i16)
        n361 = To Word Integer(number=w632) -> (16bit integer=w591:i16)
        n362 = property on="Testing area" class="Pict"() -> ("Width"=w589:u32, "Height"=w553:u32)  [unwired: 2 in, 2 out]
        n363 = call "Extract Circle Information.vi"("Circle Data"=w664) -> ("Circle x and y"=w592:cluster{"Pos. X":i32, "Pos. Y":i32})  [unwired: 1 out]
        n364 = Unbundle By Name(w592) -> ("Pos. X"=w597:i32, "Pos. Y"=w598:i32)
        n365 = Divide(x=w597, y=w591) -> (x/y=w596:dbl)
        n366 = Divide(x=w598, y=w590) -> (x/y=w595:dbl)
        n367 = call "Create Circle on Image Center.vi"("X Resolution"=w589, "Y Resolution"=w553) -> ("circle center"=w641:cluster{dbl, dbl})
        n368 = Bundle("Circle width"="Circle width", "Circle style"="Circle style") -> (w634:T21)  [unwired: 1 in]
        n369 = Multiply(x=w595, y=w553) -> (x*y=w593:dbl)
        n370 = Multiply(x=w596, y=w589) -> (x*y=w594:dbl)
        n371 = Bundle(cluster=w592, "Pos. X"=w594, "Pos. Y"=w593) -> (w562:cluster{"Pos. X":i32, "Pos. Y":i32})
        n372 = call "Empty Picture"() -> ("empty picture"=w647:picture)
        n373 = Divide(x=w589, y=w631) -> (x/y=w549:dbl)
        n374 = Divide(x=w553, y=w631) -> (x/y=w548:dbl)
        n375 = call <vilib>:"Draw Circle by Radius.vi"("pen"=w634, "color(black)"="exterior color", "fill?(F)"=w640, "pixel center"=w641, "radius"="exterior circle", "picture"=w647) -> ("new picture"=w649:picture)  [unwired: 5 in]
        n376 = To Word Integer(number=w549) -> (16bit integer=w556:i16)
        n377 = To Word Integer(number=w548) -> (16bit integer=w559:i16)
        n378 = Bundle("Circle width"="Circle width", "Style"=T2."Solid") -> (w637:T22)  [unwired: 1 in]
        n379 = call "Create bounding rectangle based on center.vi"("x center"=w556, "y center"=w559, "distance from x/y center"=i16 50) -> ("bounding rectangle coordinates"=w582:cluster{i16, i16, i16, i16})
        n380 = call <vilib>:"Draw Circle by Radius.vi"("pen"=w634, "color(black)"="middle color", "fill?(F)"=w640, "pixel center"=w641, "radius"="middle circle", "picture"=w649) -> ("new picture"=w648:picture)  [unwired: 5 in]
        n381 = Bundle(w556, w559) -> (w604:cluster{i16, i16})  [unwired: 1 in]
        n382 = call <vilib>:"Draw Circle by Radius.vi"("pen"=w637, "color(black)"="interior color", "fill?(F)"="fill static indicator", "pixel center"=w641, "radius"="interior circle", "picture"=w648) -> ("new picture"=w609:picture)  [unwired: 5 in]
        n383 = call "calculate angles.vi"("Midpoint x and y"=w604, "point"=w562) -> ("angle (degrees)"=w605:dbl)
        n384 = call <vilib>:"Draw Circle by Radius.vi"("color(black)"="center color", "fill?(F)"=w560, "pixel center"=w604, "radius"=w602, "picture"=w609) -> ("new picture"=w599:picture)  [unwired: 6 in]
        n385 = control-ref of="exterior circle"() -> (w652:refnum<vi>)
        n386 = control-ref of="middle circle"() -> (w650:refnum<vi>)
        n387 = control-ref of="interior circle"() -> (w651:refnum<vi>)
        n388 = Unbundle(w582) -> (w585:i16, w586:i16, w584:i16, w583:i16)
        n389 = To Word Integer(number=w605) -> (16bit integer=w580:i16)
        n390 = To Word Integer(number=w553) -> (16bit integer=w552:i16)
        n391 = call "Hold knobs.vi"("interior circle"=w651, "middle circle"=w650, "exterior circle"=w652) -> ()
        n392 = Bundle(cluster=w582, w585, w583, w584, w586) -> (w581:cluster{i16, i16, i16, i16})
        n393 = call <vilib>:"Draw Arc.vi"("picture"=w599, "start angle[degrees]"=i16 90, "rect"=w581, "fill?(F)"=FALSE, "color(black)"="center color", "arc size[degrees]"=w580, "pen"=T19 {"Width"=3, "Style"=enum."Solid"}) -> ("new picture"=w607:picture)  [unwired: 2 in]
        n394 = call <vilib>:"Move Pen.vi"("absolute coordinates?(T)"=w560, "new position"=w604, "picture"=w607) -> ("new picture"=w608:picture)  [unwired: 2 in]
        n395 = call <vilib>:"Draw Line.vi"("picture"=w608, "end point"=w562, "absolute coordinates?(T)"=w560, "color(black)"="center color") -> ("new picture"=w606:picture)  [unwired: 5 in]
        n396 = Decrement(x=w556) -> (x-1=w557:i16)
        n397 = Increment(x=w556) -> (x+1=w555:i16)
        n398 = Negate(x=w605) -> (-x=w558:dbl)
        n399 = call <vilib>:"Draw Circle by Radius.vi"("color(black)"="dot color", "fill?(F)"=w560, "pixel center"=w562, "radius"=w602, "picture"=w606) -> ("new picture"=w564:picture)  [unwired: 6 in]
        n400 = Bundle(w557, "Width"=i16 0, w555, w552) -> (w554:cluster{i16, "Width":i16, i16, i16})  [unwired: 1 in]
        n401 = call "Find Distance Between Points.vi"("position 2"=w604, "position 1"=w562) -> ("distance"=w610:dbl)
        n402 = call <vilib>:"Draw Rect.vi"("picture"=w564, "rect"=w554, "fill?(F)"=w560, "color(black)"="center color") -> ("new picture"=w545:picture)  [unwired: 5 in]
        n403 = property on="exterior circle" class="Knob (strict)"() -> ("Value"=w625:i16)  [unwired: 2 in, 2 out]
        n404 = property on="middle circle" class="Knob (strict)"() -> ("Value"=w621:i16)  [unwired: 2 in, 2 out]
        n405 = property on="interior circle" class="Knob (strict)"() -> ("Value"=w626:i16)  [unwired: 2 in, 2 out]
        n406 = To Double Precision Float(number=w625) -> (double precision float=w624:dbl)
        n407 = To Double Precision Float(number=w626) -> (double precision float=w622:dbl)
        n408 = To Double Precision Float(number=w621) -> (double precision float=w623:dbl)
        n409 = Greater?(x=w610, y=w624) -> (0:w620:bool)
        "outside" <- w620
        n410 = Less Or Equal?(x=w610, y=w624) -> (x <= y?=w630:bool)
        n411 = Greater?(x=w610, y=w623) -> (0:w629:bool)
        n412 = Less Or Equal?(x=w610, y=w623) -> (x <= y?=w628:bool)
        n413 = Greater?(x=w610, y=w622) -> (0:w627:bool)
        n414 = Less Or Equal?(x=w610, y=w622) -> (x <= y?=w611:bool)
        "interior" <- w611
        n415 = And(x=w628, y=w627) -> (x .and. y?=w618:bool)
        "middle" <- w618
        n416 = And(x=w630, y=w629) -> (x .and. y?=w619:bool)
        "exterior" <- w619
        n417 = case shown="True" "record (F2)" {
          tunnel: w658 -> [w743 w784]
          tunnel: [w710 w761] -> w657
          tunnel: w656 -> [w742 w783]
          tunnel: w620 -> [w722 _]
          tunnel: w619 -> [w721 _]
          tunnel: w618 -> [w720 _]
          tunnel: w614 -> [w719 w752]
          tunnel: w613 -> [w718 w763]
          tunnel: [w716 w762] -> w612
          tunnel: w611 -> [w713 _]
          tunnel: w610 -> [w712 _]
          tunnel: w558 -> [w711 _]
          tunnel: [w709 w760] -> w572
          tunnel: [w708 w759] -> w571
          tunnel: [w707 w758] -> w569
          tunnel: [w706 w757] -> w570
          tunnel: [w705 w756] -> w565
          tunnel: [w704 w755] -> w566
          tunnel: [w703 w754] -> w567
          tunnel: [w702 w753] -> w568
          tunnel: w550 -> [w698 w749]
          tunnel: w547 -> [w699 w748]
          tunnel: [w694 w744] -> w544
          frame True {
            n418 = Build Array(w712) -> (→"distance":dbl[])
            n419 = Build Array(w711) -> (→"angles":dbl[])
            n420 = Index Array(array=w743, index #1=0 ("index"), index #2=1 ("index"), index #3=2 ("index"), index #4=3 ("index"), index #5=4 ("index")) -> (element #1=w730:refnum<class "Timer.lvclass">, element #2=w729:refnum<class "Timer.lvclass">, element #3=w728:refnum<class "Timer.lvclass">, element #4=w727:refnum<class "Timer.lvclass">, element #5=w697:refnum<class "Timer.lvclass">)
            n421 = call-dynamic "Timer data class VI - add states.vi"("Reset"=w698, "Start/Stop"=w699, "Timer in"=w697) -> ("error out"=w700:errorcluster, "Timer out"=w696:refnum<class "Timer.lvclass">)  [unwired: 7 in]
            n422 = call-dynamic "Timer data class VI - add states.vi"("Reset"=w742, "Start/Stop"=w722, "Timer in"=w730) -> ("Timer out"=w741:refnum<class "Timer.lvclass">)  [unwired: 7 in, 1 out]
            n423 = call-dynamic "Timer data class VI - add states.vi"("Reset"=w742, "Start/Stop"=w721, "Timer in"=w729) -> ("error out"=w740:errorcluster, "Timer out"=w739:refnum<class "Timer.lvclass">)  [unwired: 7 in]
            n424 = call-dynamic "Timer data class VI - add states.vi"("Reset"=w742, "Start/Stop"=w720, "Timer in"=w728) -> ("error out"=w738:errorcluster, "Timer out"=w737:refnum<class "Timer.lvclass">)  [unwired: 7 in]
            n425 = call-dynamic "Timer data class VI - add states.vi"("Reset"=w742, "Start/Stop"=w713, "Timer in"=w727) -> ("error out"=w736:errorcluster, "Timer out"=w735:refnum<class "Timer.lvclass">)  [unwired: 7 in]
            n426 = call-dynamic "Timer data class VI - timer interface.vi"("error in (no error)"=w738, "Timer in"=w737) -> ("counter"=w703:i8, "time"=w707:string, "Timer out"=w724:refnum<class "Timer.lvclass">)  [unwired: 5 in, 2 out]
            n427 = call-dynamic "Timer data class VI - timer interface.vi"("error in (no error)"=w700, "Timer in"=w696) -> ("Timer out"=w695:refnum<class "Timer.lvclass">, "Milliseconds"=w694:u32)  [unwired: 5 in, 3 out]
            n428 = call-dynamic "Timer data class VI - timer interface.vi"("error in (no error)"=w736, "Timer in"=w735) -> ("counter"=w702:i8, "time"=w706:string, "Timer out"=w723:refnum<class "Timer.lvclass">)  [unwired: 5 in, 2 out]
            n429 = call-dynamic "Timer data class VI - timer interface.vi"("Timer in"=w741) -> ("counter"=w705:i8, "time"=w709:string, "Timer out"=w726:refnum<class "Timer.lvclass">)  [unwired: 6 in, 2 out]
            n430 = call-dynamic "Timer data class VI - timer interface.vi"("error in (no error)"=w740, "Timer in"=w739) -> ("counter"=w704:i8, "time"=w708:string, "Timer out"=w725:refnum<class "Timer.lvclass">)  [unwired: 5 in, 2 out]
            n431 = call-dynamic "Waveform data class VI - add waveform data.vi"("Waveform data in"=w719, "angle"=w711, "displacement"=w712) -> ("Waveform data out"=w717:refnum<class "Waveform data.lvclass">)  [unwired: 11 in, 1 out]
            n432 = Build Array(w717, w718) -> (w716:refnum<class "Waveform data.lvclass">[])
            n433 = Build Array(w726, w725, w724, w723, w695) -> (w710:refnum<class "Timer.lvclass">[])
            "distance" <- w712
            "angles" <- w711
          }
          frame False {
            n434 = Index Array(array=w784, index #1=0 ("index"), index #2=1 ("index"), index #3=2 ("index"), index #4=3 ("index"), index #5=4 ("index")) -> (element #1=w771:refnum<class "Timer.lvclass">, element #2=w770:refnum<class "Timer.lvclass">, element #3=w769:refnum<class "Timer.lvclass">, element #4=w768:refnum<class "Timer.lvclass">, element #5=w747:refnum<class "Timer.lvclass">)
            n435 = call-dynamic "Timer data class VI - add states.vi"("Reset"=w783, "Timer in"=w771) -> ("Timer out"=w782:refnum<class "Timer.lvclass">)  [unwired: 8 in, 1 out]
            n436 = call-dynamic "Timer data class VI - add states.vi"("Reset"=w783, "Timer in"=w770) -> ("error out"=w781:errorcluster, "Timer out"=w780:refnum<class "Timer.lvclass">)  [unwired: 8 in]
            n437 = call-dynamic "Timer data class VI - add states.vi"("Reset"=w783, "Timer in"=w769) -> ("error out"=w779:errorcluster, "Timer out"=w778:refnum<class "Timer.lvclass">)  [unwired: 8 in]
            n438 = call-dynamic "Timer data class VI - add states.vi"("Reset"=w783, "Timer in"=w768) -> ("error out"=w777:errorcluster, "Timer out"=w776:refnum<class "Timer.lvclass">)  [unwired: 8 in]
            n439 = call-dynamic "Timer data class VI - add states.vi"("Reset"=w749, "Start/Stop"=w748, "Timer in"=w747) -> ("error out"=w750:errorcluster, "Timer out"=w746:refnum<class "Timer.lvclass">)  [unwired: 7 in]
            n440 = call-dynamic "Timer data class VI - timer interface.vi"("error in (no error)"=w779, "Timer in"=w778) -> ("counter"=w754:i8, "time"=w758:string, "Timer out"=w765:refnum<class "Timer.lvclass">)  [unwired: 5 in, 2 out]
            n441 = call-dynamic "Timer data class VI - timer interface.vi"("error in (no error)"=w777, "Timer in"=w776) -> ("counter"=w753:i8, "time"=w757:string, "Timer out"=w764:refnum<class "Timer.lvclass">)  [unwired: 5 in, 2 out]
            n442 = call-dynamic "Timer data class VI - timer interface.vi"("Timer in"=w782) -> ("counter"=w756:i8, "time"=w760:string, "Timer out"=w767:refnum<class "Timer.lvclass">)  [unwired: 6 in, 2 out]
            n443 = call-dynamic "Timer data class VI - timer interface.vi"("error in (no error)"=w750, "Timer in"=w746) -> ("Timer out"=w745:refnum<class "Timer.lvclass">, "Milliseconds"=w744:u32)  [unwired: 5 in, 3 out]
            n444 = call-dynamic "Timer data class VI - timer interface.vi"("error in (no error)"=w781, "Timer in"=w780) -> ("counter"=w755:i8, "time"=w759:string, "Timer out"=w766:refnum<class "Timer.lvclass">)  [unwired: 5 in, 2 out]
            n445 = Build Array(w752, w763) -> (w762:refnum<class "Waveform data.lvclass">[])
            n446 = Build Array(w767, w766, w765, w764, w745) -> (w761:refnum<class "Timer.lvclass">[])
          }
        }
        "outer counter" <- w565
        "exterior counter" <- w566
        "middle counter" <- w567
        "inner counter" <- w568
        "Time outside circles" <- w572
        "Time in exterior circle" <- w571
        "Time in middle circle" <- w569
        "Time in inner circle" <- w570
        n447 = case shown="True" w547 {
          tunnel: w544 -> [_ w685]
          tunnel: w549 -> [_ w667]
          tunnel: w548 -> [_ w666]
          tunnel: [w665 w673] -> w546
          tunnel: w545 -> [w665 w672]
          frame False {
          }
          frame True {
            n448 = To Double Precision Float(number=w685) -> (double precision float=w671:dbl)
            n449 = Compound Arithmetic op=MULTIPLY(0.01, "speed", w671) -> (w688:dbl)
            n450 = Divide(x=w688, y=180.0) -> (x/y=w691:dbl)
            n451 = Multiply(x=w691, y=3.141592653589793) -> (x*y=w689:dbl)
            n452 = Sine & Cosine(0:w689) -> (1:w683:dbl, 2:w682:dbl)
            n453 = To Double Precision Float(number="radius out") -> (double precision float=w684:dbl)
            n454 = Multiply(x=w684, y=w683) -> (x*y=w680:dbl)
            n455 = Multiply(x=w684, y=w682) -> (x*y=w681:dbl)
            n456 = Add(x=w667, y=w680) -> (x+y=w676:dbl)
            n457 = Add(x=w666, y=w681) -> (x+y=w675:dbl)
            n458 = To Unsigned Long Integer(number=w676) -> (unsigned 32bit integer=w670:u32)
            n459 = To Unsigned Long Integer(number=w675) -> (unsigned 32bit integer=w669:u32)
            n460 = property on="Testing area" class="Pict"() -> ("Draw Area Size"=w674:T23)  [unwired: 2 in, 2 out]
            n461 = Bundle By Name(cluster=w674, "Width"=w670, "Height"=w669) -> (w678:T23)
            n462 = call <vilib>:"Draw Circle by Radius.vi"("color(black)"="indicator color", "fill?(F)"=TRUE, "pixel center"=w678, "radius"="indicator radius", "picture"=w672) -> ("new picture"=w673:picture)  [unwired: 6 in]
          }
        }
        "Testing area" <- w546
        n463 = case shown="True" w660 {
          tunnel: [Interface_states."Record" ("Enum") Interface_states."Idle" ("Enum")] -> w659
          frame False {
          }
          frame True {
          }
        }
      }
      frame "Reset" {
      }
      frame "Analyze" {
        w864 = enum32{"none", "unbiased", "biased"}."none" ("normalization")
        n464 = case shown="\"Testing Page\"" w887 {
          tunnel: [1 0] -> w888
          tunnel: [0 1] -> w892
          frame "Import .avi File", Default {
          }
          frame "Testing Page" {
          }
        }
        n465 = Index Array(array=w900, index #1=w888, index #2=w892) -> (element #1=w901:refnum<class "Waveform data.lvclass">, element #2=w889:refnum<class "Waveform data.lvclass">)
        n466 = call-dynamic "Waveform data class VI - retrieve waveform data.vi"("Waveform data in"=w901) -> ("Waveform data out"=w907:refnum<class "Waveform data.lvclass">, "angles"=w869:dbl[], "displacement"=w874:dbl[])  [unwired: 11 in, 1 out]
        n467 = case shown="\"Testing Page\"" w887 {
          tunnel: w874 -> [w922 w927]
          tunnel: w869 -> [w923 w928]
          tunnel: [w921 w928] -> w897
          tunnel: [w920 w927] -> w896
          tunnel: [w919 w926] -> w894
          tunnel: [w917 w925] -> w893
          frame "Import .avi File", Default {
            n468 = property on="Slide" class="Slide (strict)"() -> ("Value"=w916:cluster{u32, u32, u32})  [unwired: 2 in, 2 out]
            n469 = local read "FPS"() -> (w918:u32)
            n470 = Unbundle(w916) -> (w924:u32, w915:u32)  [unwired: 1 out]
            n471 = To Double Precision Float(number=w918) -> (double precision float=w917:dbl)
            n472 = Subtract(x=w924, y=w915) -> (x-y=w919:u32)
            n473 = Array Subset(array=w923, index=w915, length=w919) -> (w921:dbl[])
            n474 = Array Subset(array=w922, index=w915, length=w919) -> (w920:dbl[])
          }
          frame "Testing Page" {
            n475 = local read "Image Number"() -> (w926:u32)
            n476 = local read "Frame Rate"() -> (w925:dbl)
          }
        }
        n477 = To Double Precision Float(number=w896) -> (double precision float=w895:dbl[])
        n478 = call "Remove DC Offset through Scaling.vi"("unscaled array"=w895) -> ("scaled array"=w883:dbl[])
        n479 = call "Remove DC Offset through Scaling.vi"("unscaled array"=w897) -> ("scaled array"=w875:dbl[])
        n480 = property on="Tab Control" class="TabCtl (strict)"("Val(Sgnl)"=T4."Analysis (FFT/Statistics)" ("Value (Signaling)")) -> ()  [unwired: 2 in, 2 out]
        n481 = call "FFT Conversion.vi"("Number of Channels"=w894, "Frame Rate"=w893, "input array"=w875) -> ("FFT"=w906:dbl[])  [unwired: 1 out]
        "FFT theta" <- w906
        n482 = call "FFT Conversion.vi"("Number of Channels"=w894, "Frame Rate"=w893, "input array"=w883) -> ("X scale factor"=w886:dbl, "FFT"=w905:dbl[])
        "FFT displacement" <- w905
        n483 = Array Size(array=w906) -> (size(s)=→"number of channels":i32)
        n484 = property on="FFT theta" class="WFGraph (strict)"("XScale.Multiplier"=w886) -> ()  [unwired: 2 in, 2 out]
        n485 = property on="FFT displacement" class="WFGraph (strict)"("XScale.Multiplier"=w886) -> ()  [unwired: 2 in, 2 out]
        n486 = call-dynamic "Waveform data class VI - add FFT data.vi"("Waveform data in"=w907, "Angles FFT"=w906, "displacement FFT"=w905) -> ("Waveform data out"=w890:refnum<class "Waveform data.lvclass">)  [unwired: 11 in, 1 out]
        n487 = call <vilib>:"General Histogram.vi"("X"=w869) -> ("Histogram Graph"=→"theta histogram":T12)  [unwired: 10 in, 4 out]
        n488 = call-poly <vilib>:"AutoCorrelation.vi"("normalization"=w864, "X"=w869) -> ("Rxx"=→"autocorrelation theta":dbl[])  [unwired: 8 in, 1 out]
        n489 = call <vilib>:"Std Deviation and Variance.vi"("X"=w869) -> ("mean"=→"theta mean":dbl, "standard deviation"=→"theta STD":dbl, "variance"=→"theta VAR":dbl)  [unwired: 1 in]
        n490 = Array Size(array=w869) -> (size(s)=w870:i32)
        n491 = Negate(x=w870) -> (-x=w871:i32)
        n492 = To Double Precision Float(number=w871) -> (double precision float=w865:dbl)
        n493 = Array Size(array=w874) -> (size(s)=w873:i32)
        n494 = call <vilib>:"General Histogram.vi"("X"=w874) -> ("Histogram Graph"=→"displacement histogram":T12)  [unwired: 10 in, 4 out]
        n495 = call-poly <vilib>:"AutoCorrelation.vi"("normalization"=w864, "X"=w874) -> ("Rxx"=→"autocorrelation displacement":dbl[])  [unwired: 8 in, 1 out]
        n496 = call <vilib>:"Std Deviation and Variance.vi"("X"=w874) -> ("mean"=→"displacement mean":dbl, "standard deviation"=→"displacement STD":dbl, "variance"=→"displacement VAR":dbl)  [unwired: 1 in]
        n497 = Negate(x=w873) -> (-x=w872:i32)
        n498 = property on="autocorrelation theta" class="WFGraph (strict)"("XScale.Offset"=w865) -> ()  [unwired: 2 in, 2 out]
        n499 = To Double Precision Float(number=w872) -> (double precision float=w867:dbl)
        n500 = property on="autocorrelation displacement" class="WFGraph (strict)"("XScale.Offset"=w867) -> ()  [unwired: 2 in, 2 out]
        n501 = case shown="\"Testing Page\"" w887 {
          tunnel: [w909 w914] -> w891
          tunnel: w890 -> [w910 w913]
          tunnel: w889 -> [w911 w912]
          frame "Import .avi File", Default {
            n502 = Build Array(w911, w910) -> (w909:refnum<class "Waveform data.lvclass">[])
          }
          frame "Testing Page" {
            n503 = Build Array(w913, w912) -> (w914:refnum<class "Waveform data.lvclass">[])
          }
        }
      }
      frame "Save" {
        n504 = case shown="\"Analysis (FFT/Statistics)\"" w935 {
          tunnel: [1 0 0 0] -> w938
          tunnel: [0 1 1 1] -> w934
          frame "Import .avi File", Default {
          }
          frame "Testing Page" {
          }
          frame "Image Configuration" {
          }
          frame "Analysis (FFT/Statistics)" {
          }
        }
        n505 = Index Array(array=w937, index #1=w938, index #2=w934) -> (element #1=w936:refnum<class "Waveform data.lvclass">)  [unwired: 1 out]
        n506 = while {
          tunnel: w936 -> [w955]
          tunnel: w935 -> [w953]
          tunnel: w933 -> [w951]
          stop <- w954 stop-if-true
          n507 = event shown="[2] \"Optical FFTs\": Value Change" {
            selector: _ -> [_ _ _ _]
            dyn-events: _ -> [_ _ _ _]
            timeout: _ -> [_ _ _ _]
            tunnel: w955 -> [_ _ w1036 w1083]
            tunnel: [_ w956 w1035 w1082] -> w952
            tunnel: w953 -> [_ _ w1034 w1081]
            tunnel: w951 -> [_ _ w1021 w1068]
            event Timeout {
              n508 = event-data() -> ()  [unwired: 1 in, 2 out]
            }
            event "Save Config": Value Change {
              n509 = event-data() -> ("NewVal"=w957:bool)  [unwired: 1 in, 4 out]
              n510 = case shown="True" w957 {
                tunnel: [_ w1009] -> w956
                frame False {
                }
                frame True {
                  n511 = property on="file path" class="Path"() -> ("Value"=w1002:path)  [unwired: 2 in, 2 out]
                  n512 = property on="Replace Value - video player" class="DigNum (strict)"() -> ("Value"=w1001:sgl)  [unwired: 2 in, 2 out]
                  n513 = property on="Keep/Replace - video player" class="Bool (strict)"() -> ("Value"=w1000:bool)  [unwired: 2 in, 2 out]
                  n514 = property on="Range - video player" class="Clust (strict)"() -> ("Value"=w999:cluster{"Lower value":sgl, "Upper value":sgl})  [unwired: 2 in, 2 out]
                  n515 = property on="Toggle Controls - video player" class="Clust (strict)"() -> ("Value"=w998:T7)  [unwired: 2 in, 2 out]
                  n516 = property on="Connectivity 4/8: 4" class="Bool (strict)"() -> ("Value"=w997:bool)  [unwired: 2 in, 2 out]
                  n517 = property on="Connectivity 4/8: 5" class="Bool (strict)"() -> ("Value"=w996:bool)  [unwired: 2 in, 2 out]
                  n518 = property on="Square/Hexagon: video player" class="Bool (strict)"() -> ("Value"=w995:bool)  [unwired: 2 in, 2 out]
                  n519 = property on="Number of Erosion: video player" class="DigNum (strict)"() -> ("Value"=w994:i32)  [unwired: 2 in, 2 out]
                  n520 = property on="Low Pass/High Pass: video player" class="Bool (strict)"() -> ("Value"=w993:bool)  [unwired: 2 in, 2 out]
                  n521 = property on="ROI Descriptor - video player" class="Clust (strict)"() -> ("Value"=w992:T15)  [unwired: 2 in, 2 out]
                  n522 = property on="Connectivity 4/8: 6" class="Bool (strict)"() -> ("Value"=w991:bool)  [unwired: 2 in, 2 out]
                  n523 = property on="Selection Values - video player" class="Arr (strict)"() -> ("Value"=w990:T10)  [unwired: 2 in, 2 out]
                  n524 = property on="Keep/Remove Particles - video player" class="Bool (strict)"() -> ("Value"=w989:bool)  [unwired: 2 in, 2 out]
                  n525 = property on="center color" class="ColBox"() -> ("Value"=w967:u32)  [unwired: 2 in, 2 out]
                  n526 = property on="dot color" class="ColBox"() -> ("Value"=w968:u32)  [unwired: 2 in, 2 out]
                  n527 = property on="Max Radius - video player" class="DigNum (strict)"() -> ("Value"=w969:sgl)  [unwired: 2 in, 2 out]
                  n528 = property on="Min Radius - video player" class="DigNum (strict)"() -> ("Value"=w970:sgl)  [unwired: 2 in, 2 out]
                  n529 = property on="exterior color" class="ColBox"() -> ("Value"=w961:u32)  [unwired: 2 in, 2 out]
                  n530 = property on="middle color" class="ColBox"() -> ("Value"=w962:u32)  [unwired: 2 in, 2 out]
                  n531 = property on="interior color" class="ColBox"() -> ("Value"=w963:u32)  [unwired: 2 in, 2 out]
                  n532 = property on="exterior circle" class="Knob (strict)"() -> ("Value"=w964:i16)  [unwired: 2 in, 2 out]
                  n533 = property on="middle circle" class="Knob (strict)"() -> ("Value"=w965:i16)  [unwired: 2 in, 2 out]
                  n534 = property on="interior circle" class="Knob (strict)"() -> ("Value"=w966:i16)  [unwired: 2 in, 2 out]
                  n535 = property on="Circle width" class="Knob (strict)"() -> ("Value"=w960:i8)  [unwired: 2 in, 2 out]
                  n536 = property on="Circle style" class="Enum (strict)"() -> ("Value"=w959:T2)  [unwired: 2 in, 2 out]
                  n537 = property on="fill static indicator" class="Bool (strict)"() -> ("Value"=w958:bool)  [unwired: 2 in, 2 out]
                  n538 = property on="Replace Value" class="DigNum (strict)"() -> ("Value"=w971:sgl)  [unwired: 2 in, 2 out]
                  n539 = property on="Keep/Replace" class="Bool (strict)"() -> ("Value"=w972:bool)  [unwired: 2 in, 2 out]
                  n540 = property on="Range" class="Clust (strict)"() -> ("Value"=w973:cluster{"Lower value":sgl, "Upper value":sgl})  [unwired: 2 in, 2 out]
                  n541 = property on="Image Type" class="Ring (strict)"() -> ("Value"=w974:u32)  [unwired: 2 in, 2 out]
                  n542 = property on="Toggle Controls" class="Clust (strict)"() -> ("Value"=w975:T7)  [unwired: 2 in, 2 out]
                  n543 = property on="Connectivity 4/8: 3" class="Bool (strict)"() -> ("Value"=w976:bool)  [unwired: 2 in, 2 out]
                  n544 = property on="Connectivity 4/8: 2" class="Bool (strict)"() -> ("Value"=w977:bool)  [unwired: 2 in, 2 out]
                  n545 = property on="Square/Hexagon:" class="Bool (strict)"() -> ("Value"=w978:bool)  [unwired: 2 in, 2 out]
                  n546 = property on="Number of Erosion:" class="DigNum (strict)"() -> ("Value"=w979:i32)  [unwired: 2 in, 2 out]
                  n547 = property on="Low Pass/High Pass:" class="Bool (strict)"() -> ("Value"=w980:bool)  [unwired: 2 in, 2 out]
                  n548 = property on="ROI Descriptor" class="Clust (strict)"() -> ("Value"=w981:T15)  [unwired: 2 in, 2 out]
                  n549 = property on="Connectivity 4/8:" class="Bool (strict)"() -> ("Value"=w982:bool)  [unwired: 2 in, 2 out]
                  n550 = property on="Selection Values" class="Arr (strict)"() -> ("Value"=w983:T10)  [unwired: 2 in, 2 out]
                  n551 = property on="Keep/Remove Particles" class="Bool (strict)"() -> ("Value"=w988:bool)  [unwired: 2 in, 2 out]
                  n552 = property on="FFT Filename?" class="Path"() -> ("Value"=w987:path)  [unwired: 2 in, 2 out]
                  n553 = property on="Percent (%)" class="DigNum (strict)"() -> ("Value"=w986:dbl)  [unwired: 2 in, 2 out]
                  n554 = property on="Max Radius" class="DigNum (strict)"() -> ("Value"=w985:sgl)  [unwired: 2 in, 2 out]
                  n555 = property on="Min Radius" class="DigNum (strict)"() -> ("Value"=w984:sgl)  [unwired: 2 in, 2 out]
                  n556 = Bundle("Value"=w1002, "Value"=w1001, "Value"=w1000, "Value"=w999, "Value"=w998, "Value"=w997, "Value"=w996, "Value"=w995, "Value"=w994, "Value"=w993, "Value"=w992, "Value"=w991, "Value"=w990, "Value"=w989, "Value"=w960, "Value"=w959, "Value"=w958, "Value"=w961, "Value"=w962, "Value"=w963, "Value"=w964, "Value"=w965, "Value"=w966, "Value"=w967, "Value"=w968, "Value"=w969, "Value"=w970, "Value"=w971, "Value"=w972, "Value"=w973, "Value"=w974, "Value"=w975, "Value"=w976, "Value"=w977, "Value"=w978, "Value"=w979, "Value"=w980, "Value"=w981, "Value"=w982, "Value"=w983, "Value"=w984, "Value"=w985, "Value"=w986, "Value"=w987, "Value"=w988) -> (w1007:T24)  [unwired: 1 in]
                  n557 = Current VI's Path() -> (path=w1005:path)
                  n558 = Flatten To XML(anything=w1007) -> (xml string=w1008:string)
                  n559 = Strip Path(path=w1005) -> (stripped path=w1004:path)  [unwired: 1 out]
                  n560 = Build Path(base path=w1004, name or relative path="Settings\\config.xml") -> (appended path=w1006:path)
                  n561 = call-poly <vilib>:"Write to XML File.vi"("XML Input"=w1008, "XML File Path"=w1006) -> ()  [unwired: 7 in, 3 out]
                  n562 = One Button Dialog(message="Settings saved", button name ("OK")="OK") -> (true=w1010:bool)
                  n563 = Not(x=w1010) -> (.not. x?=w1009:bool)
                  n564 = property on="Save Config" class="Bool (strict)"("Val(Sgnl)"=w1009) -> ()  [unwired: 2 in, 2 out]
                }
              }
            }
            event "Optical FFTs": Value Change {
              n565 = event-data() -> ("NewVal"=w1037:bool)  [unwired: 1 in, 4 out]
              n566 = Index Array(array=w1021, index #1=0 ("index"), index #2=1 ("index"), index #3=2 ("index"), index #4=3 ("index")) -> (element #1=w1026:refnum<class "Timer.lvclass">, element #2=w1027:refnum<class "Timer.lvclass">, element #3=w1028:refnum<class "Timer.lvclass">, element #4=w1029:refnum<class "Timer.lvclass">)
              n567 = call-dynamic "Timer data class VI - timer interface.vi"("Timer in"=w1026) -> ("counter"=w1016:i8, "time"=w1030:string)  [unwired: 6 in, 3 out]
              n568 = call-dynamic "Timer data class VI - timer interface.vi"("Timer in"=w1027) -> ("counter"=w1015:i8, "time"=w1031:string)  [unwired: 6 in, 3 out]
              n569 = call-dynamic "Timer data class VI - timer interface.vi"("Timer in"=w1028) -> ("counter"=w1014:i8, "time"=w1032:string)  [unwired: 6 in, 3 out]
              n570 = call-dynamic "Timer data class VI - timer interface.vi"("Timer in"=w1029) -> ("counter"=w1013:i8, "time"=w1033:string)  [unwired: 6 in, 3 out]
              n571 = Build Array(w1016, w1015, w1014, w1013) -> (w1020:i8[])
              n572 = Build Array(w1030, w1031, w1032, w1033) -> (w1018:string[])
              n573 = Number To Decimal String(number=w1020) -> (decimal integer string=w1019:string[])  [unwired: 1 in]
              n574 = Build Array(w1018, w1019) -> (w1017:string[][])
              n575 = case shown="True" w1037 {
                tunnel: w1036 -> [_ w1043]
                tunnel: [_ w1044] -> w1035
                tunnel: w1034 -> [_ w1042]
                tunnel: w1017 -> [_ w1038]
                frame False {
                }
                frame True {
                  w1044 = FALSE
                  n576 = case shown="\"Analysis (FFT/Statistics)\"" w1042 {
                    tunnel: [w1052 w1055 w1057 w1059] -> w1049
                    tunnel: [w1051 w1054 w1056 w1058] -> w1045
                    frame "Import .avi File", Default {
                      n577 = local read "FPS"() -> (w1053:u32)
                      n578 = To Double Precision Float(number=w1053) -> (double precision float=w1052:dbl)
                      n579 = property on="number of channels" class="DigNum (strict)"() -> ("Value"=w1051:i32)  [unwired: 2 in, 2 out]
                    }
                    frame "Testing Page" {
                      n580 = property on="number of channels" class="DigNum (strict)"() -> ("Value"=w1054:i32)  [unwired: 2 in, 2 out]
                      n581 = property on="Frame Rate" class="DigNum (strict)"() -> ("Value"=w1055:dbl)  [unwired: 2 in, 2 out]
                    }
                    frame "Image Configuration" {
                      n582 = property on="number of channels" class="DigNum (strict)"() -> ("Value"=w1056:i32)  [unwired: 2 in, 2 out]
                      n583 = property on="Frame Rate" class="DigNum (strict)"() -> ("Value"=w1057:dbl)  [unwired: 2 in, 2 out]
                    }
                    frame "Analysis (FFT/Statistics)" {
                      n584 = property on="number of channels" class="DigNum (strict)"() -> ("Value"=w1058:i32)  [unwired: 2 in, 2 out]
                      n585 = property on="Frame Rate" class="DigNum (strict)"() -> ("Value"=w1059:dbl)  [unwired: 2 in, 2 out]
                    }
                  }
                  n586 = call-dynamic "Waveform data class VI - retrieve FFT data.vi"("Waveform data in"=w1043) -> ("Angles FFT"=w1047:dbl[], "displacement FFT"=w1046:dbl[])  [unwired: 11 in, 2 out]
                  n587 = Build Array(w1049, w1045) -> (w1050:dbl[])
                  n588 = Build Array(w1047, w1046) -> (w1041:dbl[][])
                  n589 = call "Saving as CSV files.vi"("First header"=string[][] [["Fs", "Number of channels"]] ("2D data"), "Data Parameters"=w1050, "Second header"=string[][] [["Time outside circles/counter", "Time in exterior circle/counter", "Time in middle circle/counter", "Time in inner circle/counter"]] ("2D data"), "Timer data"=w1038, "Third header"=string[][] [["Angles FFT", "X Position FFT", ""]] ("2D data"), "Curve Data"=w1041) -> ()  [unwired: 10 in]
                  n590 = property on="Optical FFTs" class="Bool (strict)"("Val(Sgnl)"=w1044) -> ()  [unwired: 2 in, 2 out]
                }
              }
            }
            event "Optical Data": Value Change {
              n591 = event-data() -> ("NewVal"=w1084:bool)  [unwired: 1 in, 4 out]
              n592 = Index Array(array=w1068, index #1=0 ("index"), index #2=1 ("index"), index #3=2 ("index"), index #4=3 ("index")) -> (element #1=w1073:refnum<class "Timer.lvclass">, element #2=w1074:refnum<class "Timer.lvclass">, element #3=w1075:refnum<class "Timer.lvclass">, element #4=w1076:refnum<class "Timer.lvclass">)
              n593 = call-dynamic "Timer data class VI - timer interface.vi"("Timer in"=w1073) -> ("counter"=w1067:i8, "time"=w1077:string)  [unwired: 6 in, 3 out]
              n594 = call-dynamic "Timer data class VI - timer interface.vi"("Timer in"=w1074) -> ("counter"=w1066:i8, "time"=w1078:string)  [unwired: 6 in, 3 out]
              n595 = call-dynamic "Timer data class VI - timer interface.vi"("Timer in"=w1075) -> ("counter"=w1065:i8, "time"=w1079:string)  [unwired: 6 in, 3 out]
              n596 = call-dynamic "Timer data class VI - timer interface.vi"("Timer in"=w1076) -> ("counter"=w1064:i8, "time"=w1080:string)  [unwired: 6 in, 3 out]
              n597 = Build Array(w1077, w1078, w1079, w1080) -> (w1062:string[])
              n598 = Build Array(w1067, w1066, w1065, w1064) -> (w1063:i8[])
              n599 = Number To Decimal String(number=w1063) -> (decimal integer string=w1060:string[])  [unwired: 1 in]
              n600 = Build Array(w1062, w1060) -> (w1061:string[][])
              n601 = case shown="True" w1084 {
                tunnel: w1083 -> [_ w1095]
                tunnel: [_ w1097] -> w1082
                tunnel: w1081 -> [_ w1094]
                tunnel: w1061 -> [_ w1085]
                frame False {
                }
                frame True {
                  w1097 = FALSE ("Value (Signaling)")
                  n602 = call-dynamic "Waveform data class VI - retrieve waveform data.vi"("Waveform data in"=w1095) -> ("angles"=w1092:dbl[], "displacement"=w1090:dbl[])  [unwired: 11 in, 2 out]
                  n603 = case shown="\"Import .avi File\", Default" w1094 {
                    tunnel: [w1100 w1112] -> w1093
                    tunnel: w1092 -> [w1105 w1111]
                    tunnel: [w1104 w1111] -> w1091
                    tunnel: w1090 -> [w1103 w1110]
                    tunnel: [w1102 w1110] -> w1089
                    frame "Import .avi File", Default {
                      n604 = property on="Slide" class="Slide (strict)"() -> ("Value"=w1108:cluster{u32, u32, u32})  [unwired: 2 in, 2 out]
                      n605 = local read "FPS"() -> (w1101:u32)
                      n606 = Unbundle(w1108) -> (w1107:u32, w1109:u32)  [unwired: 1 out]
                      n607 = To Double Precision Float(number=w1101) -> (double precision float=w1100:dbl)
                      n608 = Subtract(x=w1107, y=w1109) -> (x-y=w1106:u32)
                      n609 = Array Subset(array=w1105, index=w1109, length=w1106) -> (w1104:dbl[])
                      n610 = Array Subset(array=w1103, index=w1109, length=w1106) -> (w1102:dbl[])
                    }
                    frame "Testing Page" {
                      n611 = property on="Frame Rate" class="DigNum (strict)"() -> ("Value"=w1112:dbl)  [unwired: 2 in, 2 out]
                    }
                  }
                  n612 = Array Size(array=w1089) -> (size(s)=w1096:i32)
                  n613 = Build Array(w1093, w1096) -> (w1099:dbl[])
                  n614 = Build Array(w1091, w1089) -> (w1088:dbl[][])
                  n615 = property on="Optical Data" class="Bool (strict)"("Val(Sgnl)"=w1097) -> ()  [unwired: 2 in, 2 out]
                  n616 = call "Saving as CSV files.vi"("First header"=string[][] [["Fs", "Number of channels"]] ("2D data"), "Data Parameters"=w1099, "Second header"=string[][] [["Time outside circles/counter", "Time in exterior circle/counter", "Time in middle circle/counter", "Time in inner circle/counter"]] ("2D data"), "Timer data"=w1085, "Third header"=string[][] [["Angles", "Displacement"]] ("2D data"), "Curve Data"=w1088) -> ()  [unwired: 10 in]
                }
              }
            }
          }
          n617 = Not(x=w952) -> (.not. x?=w954:bool)
        }
      }
      frame "Open - Analyze" {
        n618 = while {
          tunnel: [w1138] -> w1117
          tunnel: w1116 -> [w1137]
          tunnel: [w1136] -> w1115
          stop <- TRUE stop-if-true
          n619 = call-dynamic "Importing FFT Data class VI - retrieve data.vi"("Imported FFT Data in"=w1137) -> ("Array 2"=w1128:dbl[][], "Array"=w1129:dbl[][], "Imported FFT Data out"=w1126:refnum<class "Imported FFT Data.lvclass">, "FFTs Table"=w1127:string[][], "Row"=w1130:i32)  [unwired: 5 in, 1 out]
          n620 = event shown="[4] \"Add FFT?\": Value Change" {
            selector: _ -> [_ _ _ _ _ _ _ _]
            dyn-events: _ -> [_ _ _ _ _ _ _ _]
            timeout: 5000 -> [_ _ _ _ _ _ _ _]
            tunnel: [w1143 w1148 w1153 w1158 w1169 w1242 w1307 w1312] -> w1124
            tunnel: [w1140 w1145 w1150 w1155 _ w1247 w1306 w1310] -> w1122
            tunnel: w1130 -> [w1140 w1145 w1150 w1155 _ w1248 w1306 w1310]
            tunnel: w1127 -> [w1142 w1147 w1152 w1157 w1187 w1245 w1308 w1313]
            tunnel: [w1142 w1147 w1152 w1157 w1188 w1244 w1308 w1313] -> w1123
            tunnel: w1128 -> [w1143 w1148 w1153 w1158 w1186 w1243 w1307 w1312]
            tunnel: w1129 -> [w1141 w1146 w1151 w1156 w1173 w1240 w1305 w1314]
            tunnel: [w1141 w1146 w1151 w1156 w1170 w1241 w1305 w1314] -> w1125
            tunnel: [Interface_states."Idle" ("Enum") Interface_states."Reset" ("Enum") Interface_states."Idle" ("Enum") Interface_states."Idle" ("Enum") Interface_states."Open - Analyze" ("Enum") Interface_states."Open - Analyze" ("Enum") Interface_states."Idle" ("Enum") Interface_states."Open - Analyze" ("Enum")] -> w1138
            event Timeout {
              n621 = event-data() -> ()  [unwired: 1 in, 2 out]
            }
            event "Reset": Value Change {
              n622 = event-data() -> ()  [unwired: 1 in, 5 out]
            }
            event "Quit": Value Change {
              n623 = event-data() -> ()  [unwired: 1 in, 5 out]
            }
            event "camera (F1)": Value Change {
              n624 = event-data() -> ()  [unwired: 1 in, 5 out]
            }
            event "Add FFT?": Value Change {
              w1179 = 0 ("disabled index (row)")
              n625 = event-data() -> ()  [unwired: 1 in, 1 out]
              n626 = Strip Path(path="FFT Filename?") -> (name=w1184:string)  [unwired: 1 out]
              n627 = Match Pattern(string=w1184, regular expression=".csv") -> (before substring=w1183:string)  [unwired: 1 in, 3 out]
              n628 = stacked-sequence {
                seq-local: [w1203 _ _] -> [_ w1210 _]
                seq-local: [_ w1208 _] -> [_ _ w1214]
                tunnel: "FFT Filename?" -> [w1201 w1211 w1218]
                tunnel: [_ _ w1217] -> w1163
                tunnel: [w1202 _ _] -> w1180
                tunnel: [_ _ w1215] -> w1182
                frame #0 {
                  w1204 = 1 ("number of rows (all:-1)")
                  w1205 = "," ("delimiter (\\t)")
                  n629 = call-poly <vilib>:"Read From Spreadsheet File.vi"("delimiter (\\t)"=w1205, "number of rows (all:-1)"=w1204, "file path (dialog if empty)"=w1201) -> ("mark after read (chars.)"=w1206:i32)  [unwired: 4 in, 4 out]
                  n630 = call-poly <vilib>:"Read From Spreadsheet File.vi"("delimiter (\\t)"=w1205, "start of read offset (chars.:0)"=w1206, "number of rows (all:-1)"=w1204, "file path (dialog if empty)"=w1201) -> ("mark after read (chars.)"=w1203:i32, "all rows"=w1202:dbl[][])  [unwired: 3 in, 3 out]
                }
                frame #1 {
                  w1213 = "," ("delimiter (\\t)")
                  n631 = call-poly <vilib>:"Read From Spreadsheet File.vi"("delimiter (\\t)"=w1213, "start of read offset (chars.:0)"=w1210, "number of rows (all:-1)"=1, "file path (dialog if empty)"=w1211) -> ("mark after read (chars.)"=w1209:i32)  [unwired: 3 in, 4 out]
                  n632 = call-poly <vilib>:"Read From Spreadsheet File.vi"("delimiter (\\t)"=w1213, "start of read offset (chars.:0)"=w1209, "number of rows (all:-1)"=2, "file path (dialog if empty)"=w1211) -> ("mark after read (chars.)"=w1208:i32)  [unwired: 3 in, 4 out]
                }
                frame #2 {
                  w1220 = "," ("delimiter (\\t)")
                  n633 = call-poly <vilib>:"Read From Spreadsheet File.vi"("delimiter (\\t)"=w1220, "start of read offset (chars.:0)"=w1214, "number of rows (all:-1)"=1, "file path (dialog if empty)"=w1218) -> ("mark after read (chars.)"=w1221:i32, "all rows"=w1215:string[][])  [unwired: 3 in, 3 out]
                  n634 = call-poly <vilib>:"Read From Spreadsheet File.vi"("delimiter (\\t)"=w1220, "transpose (no:F)"=TRUE, "start of read offset (chars.:0)"=w1221, "file path (dialog if empty)"=w1218) -> ("all rows"=w1217:dbl[][])  [unwired: 3 in, 4 out]
                }
              }
              n635 = Index Array(array=w1180, index (row) #1=w1179, index (col) #1=1 ("disabled index (col)"), index (row) #2=w1179, index (col) #2=w1179) -> (element #1=w1178:dbl, element #2=w1168:dbl)
              n636 = Array Size(array=w1163) -> (size(s)=w1181:i32[])
              n637 = Reciprocal(x=w1178) -> (1/x=w1177:dbl)
              n638 = Build Array (concatenate)(w1186, w1163) -> (w1169:dbl[][])
              n639 = Index Array(array=w1181) -> (element #1=w1174:i32)  [unwired: 2 in, 1 out]
              n640 = To Long Integer(number=w1178) -> (32bit integer=w1172:i32)
              n641 = Divide(x=w1168, y=2.0) -> (x/y=w1167:dbl)
              n642 = Multiply(x=w1177, y=w1167) -> (x*y=w1176:dbl)
              n643 = for {
                N: w1172 -> [_]
                tunnel: w1176 -> [w1200]
                tunnel: [w1198] -> w1175 mode=indexing
                i -> [w1199]
                n644 = Multiply(x=w1200, y=w1199) -> (x*y=w1198:dbl)
              }
              n645 = for {
                N: w1174 -> [_]
                tunnel: w1175 -> [w1197]
                tunnel: [w1197] -> w1162 mode=indexing
              }
              n646 = for {
                tunnel: w1163 -> [w1196] mode=indexing
                tunnel: w1162 -> [w1194] mode=indexing
                tunnel: [w1193] -> w1165 mode=indexing
                w1190 = 5 ("index")
                n647 = Array Subset(array=w1196, index=w1190) -> (w1195:dbl[])  [unwired: 1 in]
                n648 = Array Max & Min(array=w1195) -> (max index (indices)=w1191:i32)  [unwired: 3 out]
                n649 = Add(x=w1191, y=w1190) -> (x+y=w1192:i32)
                n650 = Index Array(array=w1194, index=w1192) -> (element=w1193:dbl)
              }
              n651 = Build Array (concatenate)(w1173, w1162) -> (w1170:dbl[][])
              n652 = Number To Fractional String(number=w1165, precision (6)=i16 6) -> (F-format string=w1160:string[])  [unwired: 2 in]
              n653 = for {
                N: w1174 -> [_]
                tunnel: w1183 -> [w1231]
                tunnel: [w1228] -> w1161 mode=indexing
                tunnel: w1182 -> [w1227]
                tunnel: w1160 -> [w1224]
                i -> [w1223]
                n654 = Index Array(array=w1227, index (col)=w1223) -> (element=w1226:string[])  [unwired: 1 in]
                n655 = Concatenate Strings(w1231, " - " ("string"), w1226) -> (w1229:string)
                n656 = Index Array(array=w1224, index=w1223) -> (element=w1222:string)
                n657 = Build Array(w1229, w1222, "YES" ("element")) -> (w1228:string[])
              }
              n658 = Build Array (concatenate)(w1187, w1161) -> (w1188:string[][])
            }
            event "FFTs Table": Mouse Down {
              n659 = event-data() -> ("Coords"=w1250:T25)  [unwired: 1 in, 3 out]
              n660 = invoke on="FFTs Table" class="Tbl (strict)" method="Point To Row Column"("Point"=w1250) -> ("CellPosition"=w1249:T26)  [unwired: 5 in, 5 out]
              n661 = Array Size(array=w1240) -> (size(s)=w1239:i32[])
              n662 = Unbundle By Name(w1249) -> ("Column"=w1246:i32, "Row"=w1236:i32)
              n663 = Index Array(array=w1239) -> (element=w1237:i32)  [unwired: 1 in]
              n664 = Decrement(x=w1237) -> (x-1=w1238:i32)
              n665 = Greater Or Equal To 0?(x=w1236) -> (x >= 0?=w1233:bool)
              n666 = Less Or Equal?(x=w1236, y=w1238) -> (x <= y?=w1234:bool)
              n667 = And(x=w1234, y=w1233) -> (x .and. y?=w1235:bool)
              n668 = case shown="True" w1235 {
                tunnel: w1236 -> [_ w1264]
                tunnel: w1248 -> [_ w1263]
                tunnel: [w1251 w1262] -> w1247
                tunnel: w1246 -> [w1251 w1261]
                tunnel: w1245 -> [w1252 w1260]
                tunnel: [w1252 w1259] -> w1244
                tunnel: w1243 -> [w1253 w1258]
                tunnel: [w1253 w1257] -> w1242
                tunnel: w1240 -> [w1254 w1256]
                tunnel: [w1254 w1255] -> w1241
                frame False {
                }
                frame True {
                  n669 = case shown="0, 1" w1261 {
                    tunnel: w1264 -> [w1265 w1272 w1277]
                    tunnel: w1263 -> [_ _ w1276]
                    tunnel: [_ w1272 w1277] -> w1262
                    tunnel: w1260 -> [w1271 w1274 w1293]
                    tunnel: [w1270 w1274 w1293] -> w1259
                    tunnel: w1258 -> [w1269 w1275 w1290]
                    tunnel: [w1268 w1275 w1290] -> w1257
                    tunnel: w1256 -> [w1267 w1273 w1288]
                    tunnel: [w1266 w1273 w1288] -> w1255
                    frame 2 {
                      n670 = Delete From Array(array=w1267, index (row)=w1265) -> (array with subset deleted=w1266:dbl[][])  [unwired: 2 in, 1 out]
                      n671 = Delete From Array(array=w1269, index (row)=w1265) -> (array with subset deleted=w1268:dbl[][])  [unwired: 2 in, 1 out]
                      n672 = Delete From Array(array=w1271, index (row)=w1265) -> (array with subset deleted=w1270:string[][])  [unwired: 2 in, 1 out]
                    }
                    frame Default {
                    }
                    frame 0, 1 {
                      n673 = flat-sequence {
                        tunnel: w1276 -> [w1294]
                        tunnel: w1277 -> [w1296]
                        frame #0 {
                          n674 = property on="FFT Visualizer" class="XYGraph (strict)"("Active Plot"=w1294, "Plot.Line Width"=u8 0) -> ()  [unwired: 2 in, 2 out]
                        }
                        frame #1 {
                          n675 = property on="FFT Visualizer" class="XYGraph (strict)"("Active Plot"=w1296, "Plot.Line Width"=u8 3) -> ()  [unwired: 2 in, 2 out]
                        }
                      }
                      n676 = Index Array(array=w1290, index (row)=w1277) -> (element=w1289:dbl[])  [unwired: 1 in]
                      n677 = Index Array(array=w1288, index (row)=w1277) -> (element=w1285:dbl[])  [unwired: 1 in]
                      n678 = Array Max & Min(array=w1289) -> (max value=w1292:dbl)  [unwired: 3 out]
                      n679 = Divide(x="Percent (%)", y=100.0) -> (x/y=w1291:dbl)
                      n680 = Multiply(x=w1292, y=w1291) -> (x*y=w1278:dbl)
                      n681 = call <vilib>:"Peak Detector.vi"("threshold"=w1278, "X"=w1289) -> ("Amplitudes"=w1284:dbl[], "Locations"=w1282:dbl[])  [unwired: 5 in, 3 out]
                      n682 = for {
                        tunnel: w1285 -> [w1302]
                        tunnel: w1282 -> [w1301] mode=indexing
                        tunnel: [w1299] -> w1283 mode=indexing
                        n683 = Round To Nearest(number=w1301) -> (nearest integer value=w1298:dbl)
                        n684 = Array Subset(array=w1302, index=w1298, length=1) -> (w1300:dbl[])
                        n685 = Index Array(array=w1300) -> (element=w1299:dbl)  [unwired: 1 in]
                      }
                      n686 = property on="FFT Visualizer" class="XYGraph (strict)"("Cursor.Cursor Y"=w1278) -> ()  [unwired: 2 in, 2 out]
                      n687 = Build Array(w1283, w1284) -> (w1287:dbl[][])
                      n688 = Transpose 2D Array(2D array=w1287) -> (transposed array=w1280:dbl[][])
                      n689 = Number To Fractional String(number=w1280) -> (F-format string=→"Peaks":string[][])  [unwired: 3 in]
                    }
                  }
                }
              }
            }
            event "Tab Control": Value Change {
              n690 = event-data() -> ()  [unwired: 1 in, 5 out]
            }
            event "Percent (%)": Value Change {
              n691 = event-data() -> ("NewVal"=w1315:dbl)  [unwired: 1 in, 4 out]
              n692 = Index Array(array=w1312, index (row)=w1310) -> (element=w1311:dbl[])  [unwired: 1 in]
              n693 = Array Max & Min(array=w1311) -> (max value=w1318:dbl)  [unwired: 3 out]
              n694 = Divide(x=w1315, y=100.0) -> (x/y=w1317:dbl)
              n695 = Multiply(x=w1318, y=w1317) -> (x*y=w1319:dbl)
              n696 = property on="FFT Visualizer" class="XYGraph (strict)"("Cursor.Cursor Y"=w1319) -> ()  [unwired: 2 in, 2 out]
            }
          }
          "FFTs Table" <- w1123
          n697 = call "Convert to Dynamic Data2"("2D Array"=w1125) -> ("Dynamic Data Type"=w1133:dynamicdata)  [unwired: 3 in]
          n698 = call "Convert to Dynamic Data"("2D Array"=w1124) -> ("Dynamic Data Type"=w1134:dynamicdata)  [unwired: 3 in]
          n699 = call "Build XY Graph"("Y Input"=w1134, "X Input"=w1133) -> ("XY Graph"=→"FFT Visualizer":cluster{"Y":dbl[], "Y":dbl[]}[])  [unwired: 3 in, 6 out]
          n700 = Array Max & Min(array=w1125) -> (max value=w1132:dbl)  [unwired: 3 out]
          n701 = property on="FFT Visualizer" class="XYGraph (strict)"("XScale.Maximum"=w1132) -> ()  [unwired: 2 in, 2 out]
          n702 = property on="FFT Visualizer" class="XYGraph (strict)"("XScale.Minimum"=0.0 ("X Scale.Range:Minimum")) -> ()  [unwired: 2 in, 2 out]
          n703 = call-dynamic "Importing FFT Data class VI - change data.vi"("FFTs Table"=w1123, "Row"=w1122, "Array 2"=w1124, "Array"=w1125, "Imported FFT Data in"=w1126) -> ("Imported FFT Data out"=w1136:refnum<class "Imported FFT Data.lvclass">)  [unwired: 5 in, 1 out]
        }
      }
    }
    n704 = Select(t=w61, s="Save Config", f=w62) -> (s? t:f=w60:T14)
    n705 = Select(t=w61, s="Optical Data", f=w60) -> (s? t:f=w78:T14)
    n706 = Select(t=w61, s="Optical FFTs", f=w78) -> (s? t:f=w77:T14)
  }
